vi "Pick&Place_ladder_shih_v4_temp.vi"() -> ()   [LabVIEW 2016]
uses:
  Classes/Controllers/I-O/Copy of NI-DAQ Folder/NI-DAQ.lvclass
  D:/INTT/V1/Classes/Controllers/I-O/Copy of I-O Folder/I-O.lvclass
  Classes/Controllers/Dispenser/Copy of Ultimus V2 Folder/Ultimus V2.lvclass
  <vilib>/Analysis/coordinate.llb/2D Cartesian Coordinate Rotation (Scalar).vi
  <vilib>/Utility/file.llb/Read Delimited Spreadsheet (DBL).vi
  <vilib>/Utility/file.llb/Write Delimited Spreadsheet (DBL).vi
  Classes/Controllers/Motion/Copy of Motion Folder/Motion.lvclass
  Classes/Controllers/Camera/Copy of Controller Folder/Controller.lvclass
  <vilib>/Analysis/NI_AALPro.lvlib
  Classes/Controllers/I-O/Copy of I-O Folder/I-O.lvclass
panel:
  in  "module placing offset":dbl[][](array[numeric])=[[0.0, 0.0, 0.0, 0.0], [0.0, 0.0, 0.0, 0.0]]
  out "after SR":dbl[](array[numeric])
  out "after NL":dbl[](array[numeric])
  out "S chip":dbl[](array[numeric])
  out "N chip":dbl[](array[numeric])
  in  "file path (dialog if empty) 2":path=path "C:/Users/PAGANIS/Desktop/shih cheng wei/OGP/test1-2.txt"
  out "bless from OGP !!! Center of module on stave 3":dbl[](array[numeric])
  out "bless from OGP !! measured stave size  2":dbl[](array[numeric])
  in  "Bless from OGP":bool
  out "FROM Detail !!! Center of module on stave":dbl[](array[numeric])
  out "FROM Detail !! measured stave size":dbl[](array[numeric])
  in  "Align Stave in detail":bool
  in  "check height?":bool
  in  "Uttimus presssure":i64=10
  out "Status":bool
  out "measured HDI top-left position":dbl[][](array[numeric])
  in  "HDI vacuum channel":i32=18
  in  "vacuum":bool=TRUE
  in  "HDI vacuum":bool
  out "measured stave size":dbl[](array[numeric])
  out "Stave mark":dbl[][](array[numeric])
  out "Center of module on stave":dbl[](array[numeric])
  out "Center of HDI from alignment mark":dbl[](array[numeric])
  out "Measured HDI size":dbl[][](array[numeric])
  out "module position on stave":dbl[][](array[numeric])
  in  "Default Stave dimension":dbl[](array[numeric])=[34.0, 472.0, -0.335295, -0.000320234]
  in  "Default Stave upper left mark":dbl[](array[numeric])=[584.376, 675.576, 70.9882, 0.000840064]
  out "Needle parking position":dbl[](array[numeric])
  in  "Uppler / Lower Stave":bool=TRUE
  out "Gantry current position":dbl[](array[numeric])
  in  "READ Position":bool
  in  "Needle Height Compenstation\n(glue gap)":dbl=0.33
  in  "Needle Alignment":bool
  in  "Parking position":dbl[](array[numeric])=[625.0, 625.0, 0.0, 0.01]
  in  "GOTO":bool
  in  "Default Pickup Tool Position":dbl[][](array[numeric])=[[152.226, 682.729, 36.8129, -0.0151898], [700.0, 800.0, 20.0, 0.01]]
  in  "Number of module \nto be assembled":i32=1
  in  "Default HDI alignment \nmark position":dbl[](array[numeric])=[448.322, 976.582, 74.9872, 0.000191129]
  in  "Default HDI size":dbl[](array[numeric])=[24.2437, 231.446, -0.099339, 0.000191129]
  out "# of tasks excuted":i32
  out "module on tray position":dbl[][](array[numeric])
  out "PickupTool \nCenterPosition":dbl[](array[numeric])
  in  "Inititalize":bool
  in  "Pick and place":bool
  in  "Deposit Glue":bool
  in  "Measure Pickup Tools":bool
  in  "Align Stave":bool
  out "default module position on stave":dbl[][](array[numeric])
  in  "Stop":bool
  in  "Measure HDI":bool
  # "Ladder Assembly"
  # "Lower\nmodule"
  # "Upper\nmodule"
  # "Sensor 0.32 -> 200 micron glue thickness\nChips 0.37-> 140 micron glue thickness"
  # "ACTIONS"
  # "Stave infomation"
  # "Module infomation"
  # "Pick and Place"
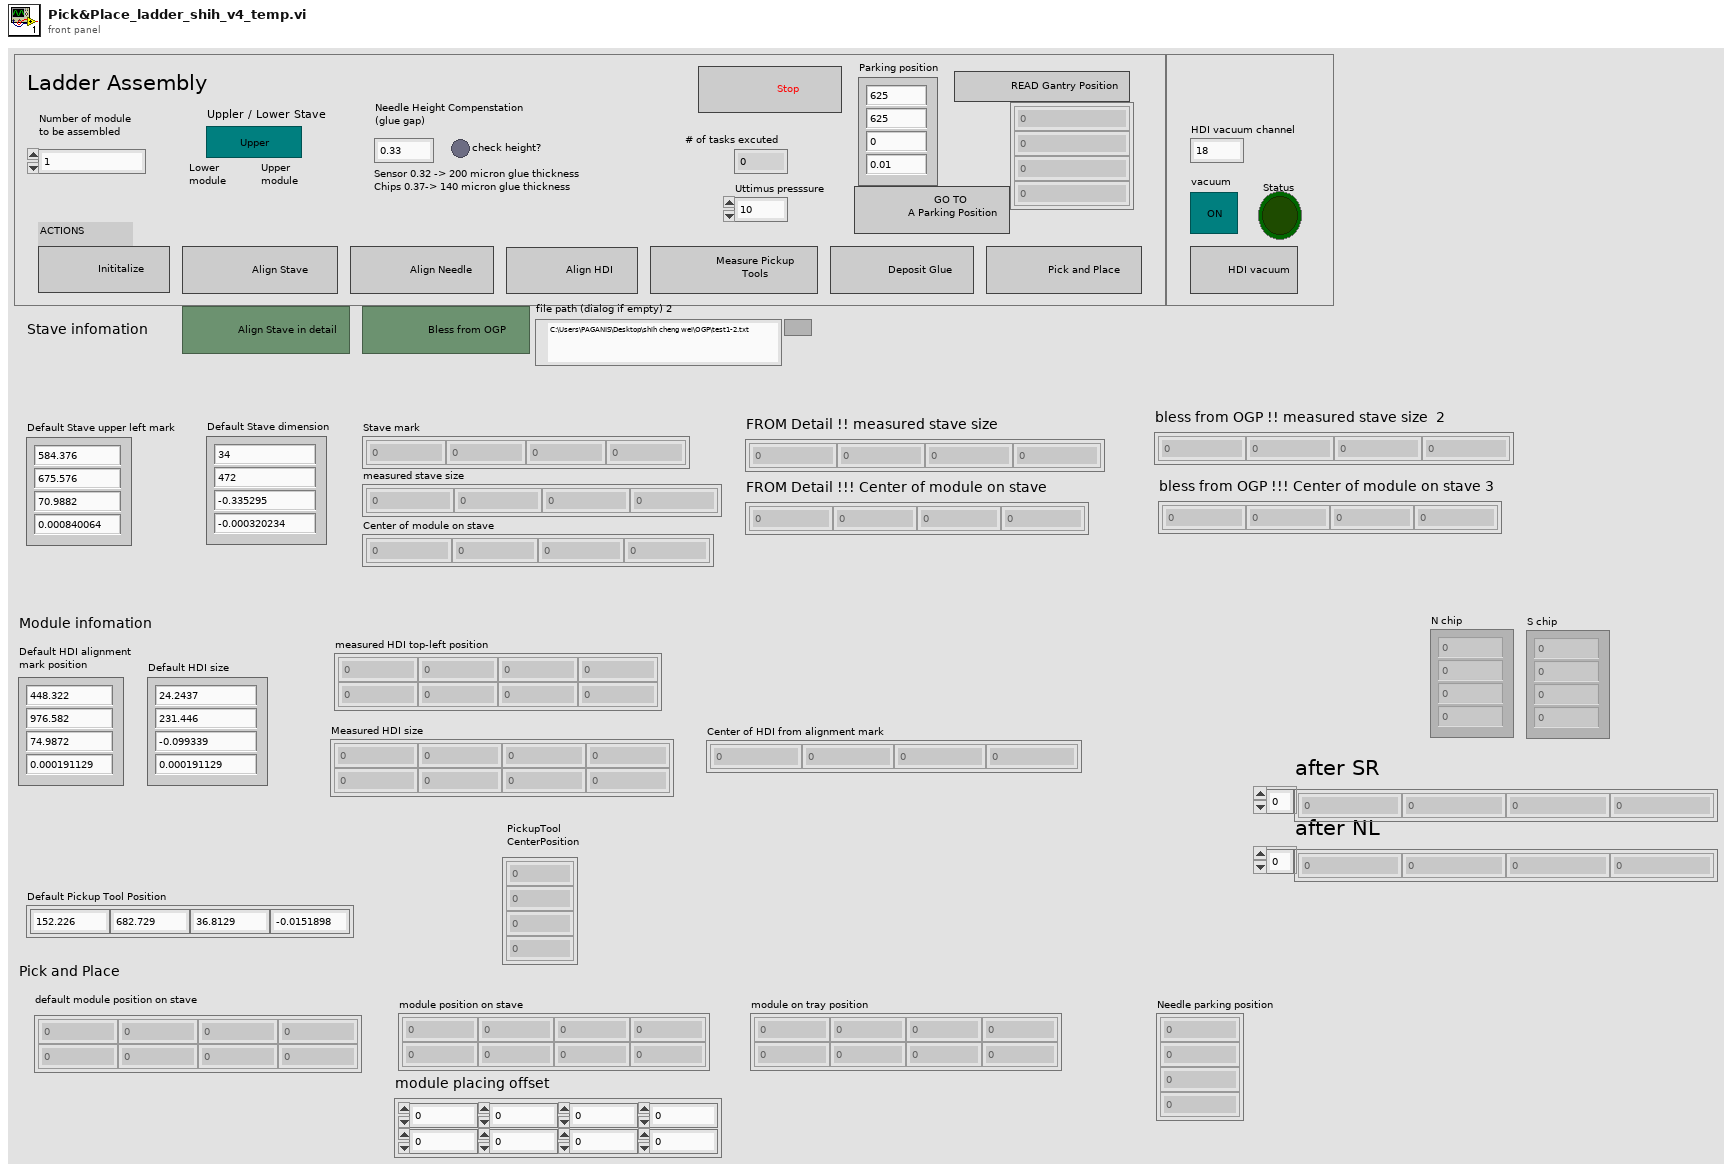
[diagram p1: front panel]
types:
  T1 = typedef "Controller.lvclass/Controllers.ctl" = cluster{"Copy of Motion.lvclass":refnum<class "Motion.lvclass">, "Copy of I-O.lvclass":refnum<class "I-O.lvclass">, "Copy of Dispenser.lvclass":refnum<class "Dispenser.lvclass">}
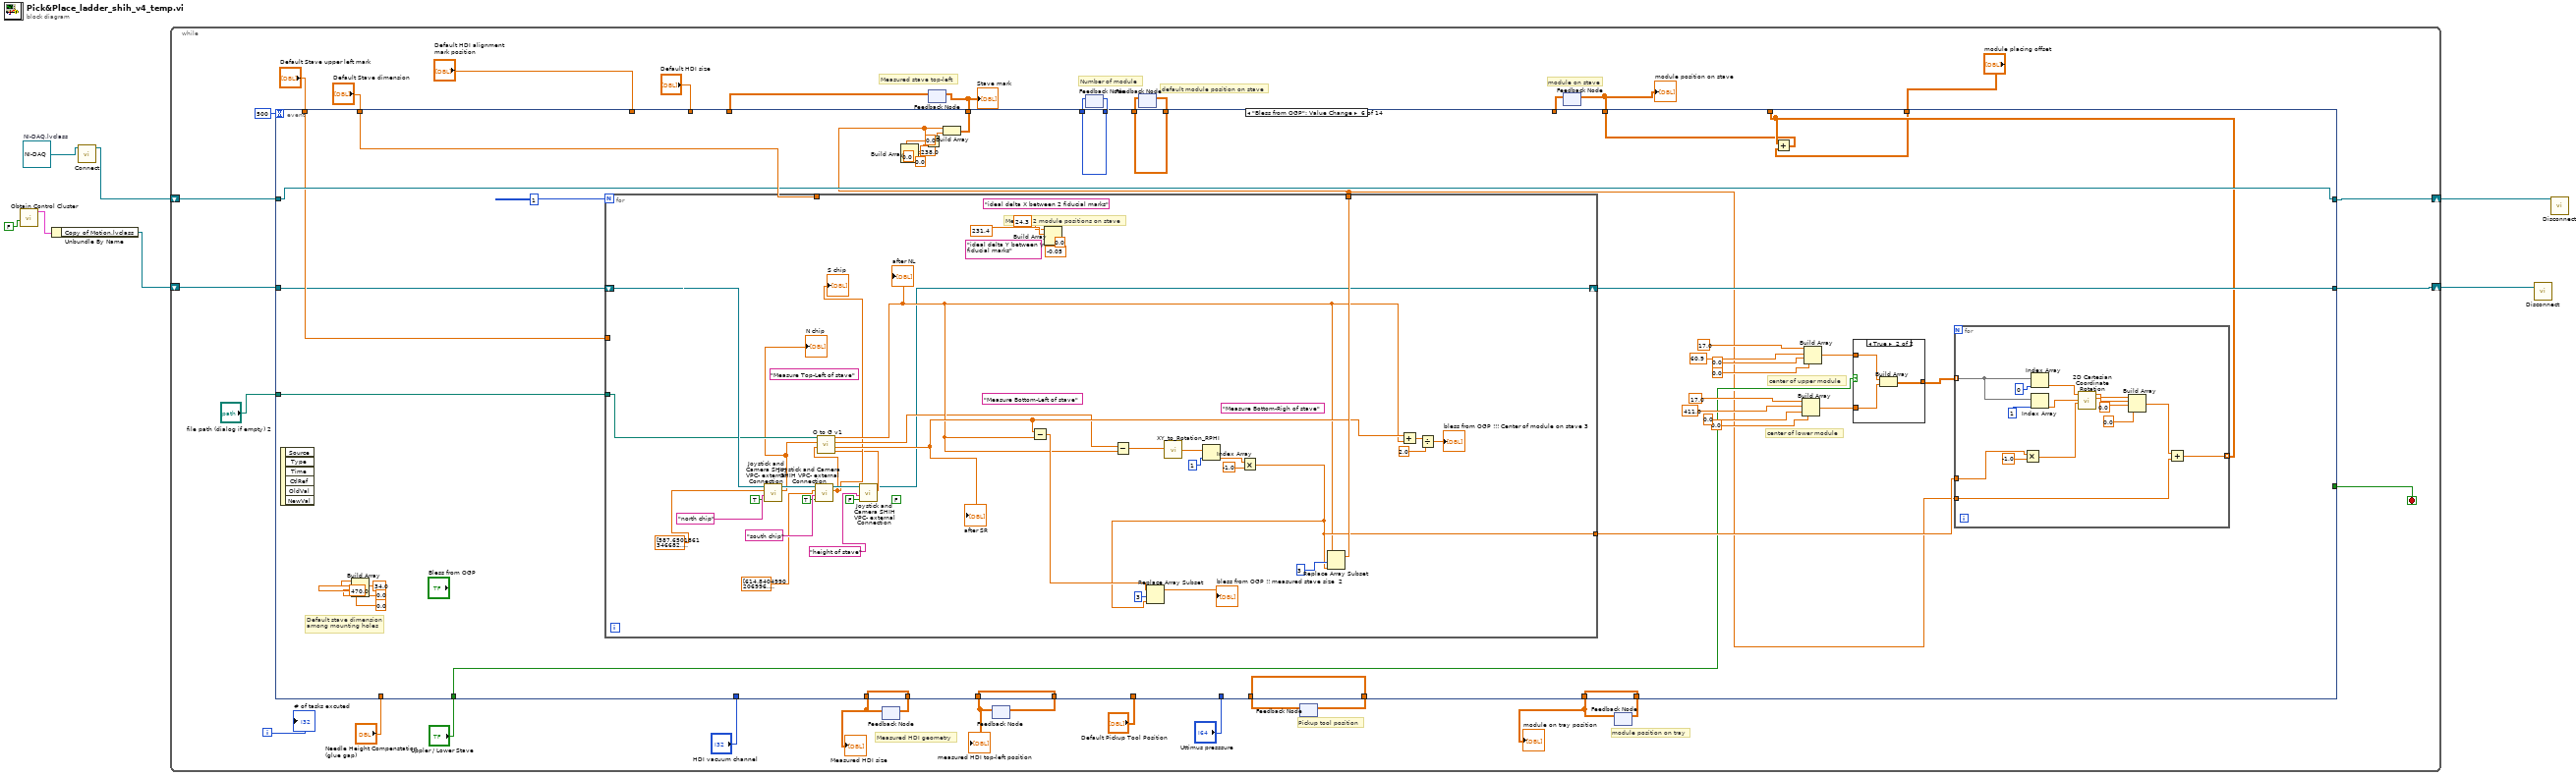
[diagram p0: block diagram]
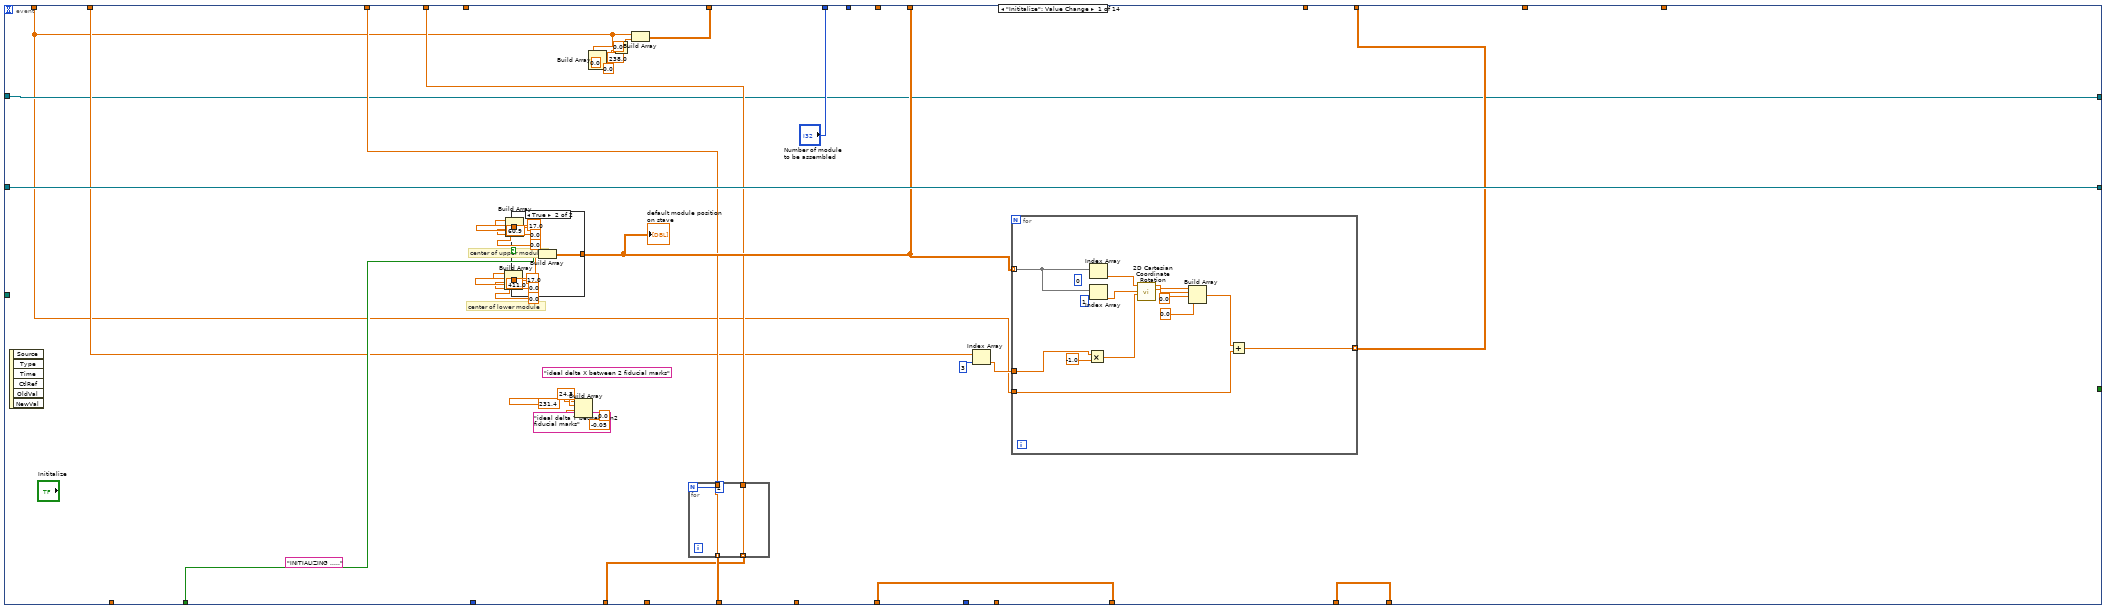
[diagram p2: hidden frame]
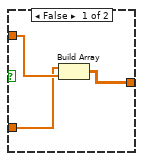
[diagram p3: hidden frame]
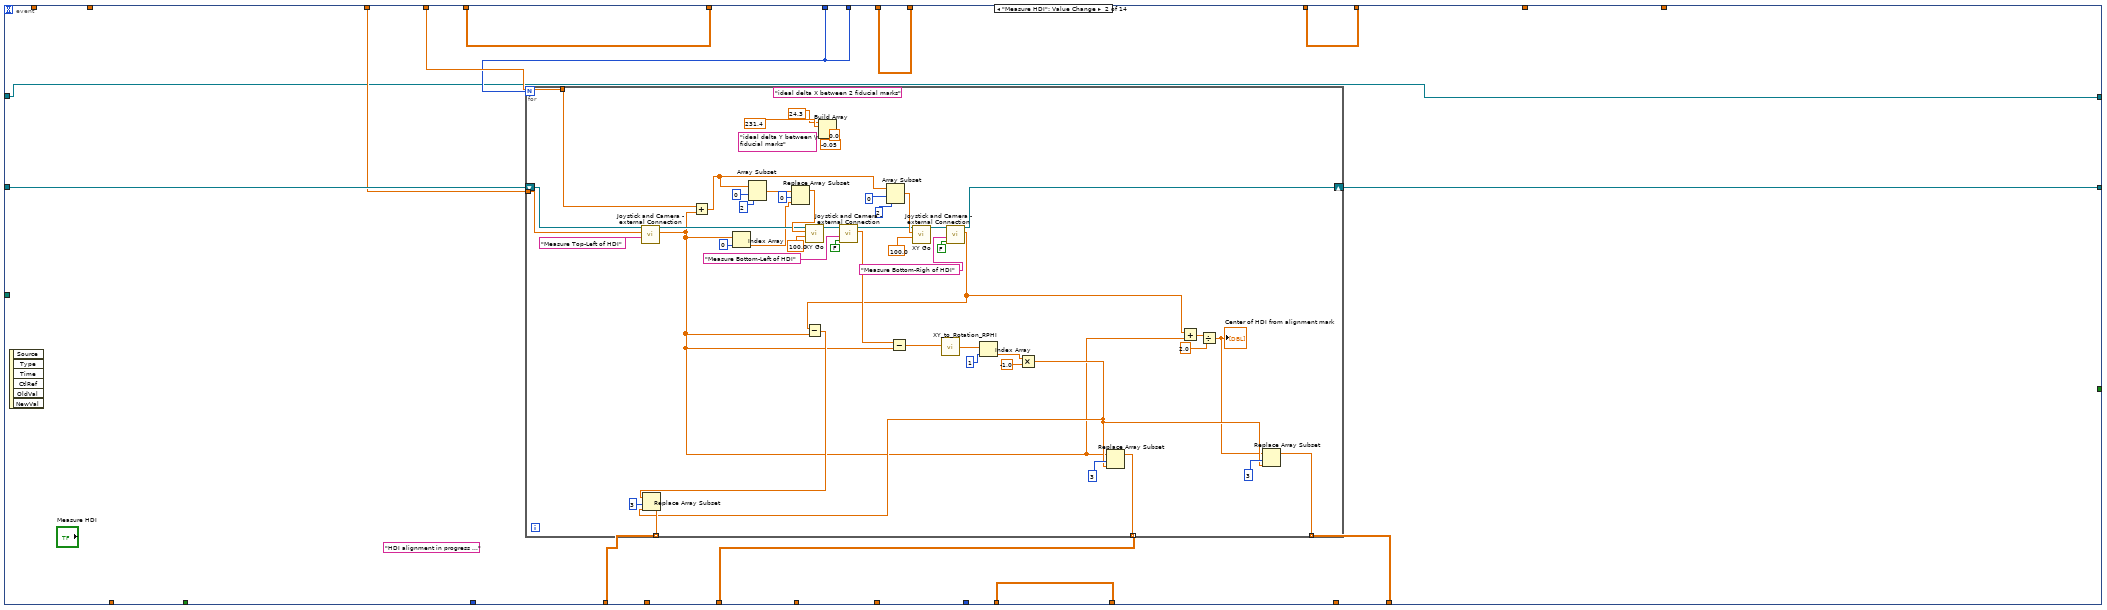
[diagram p4: hidden frame]
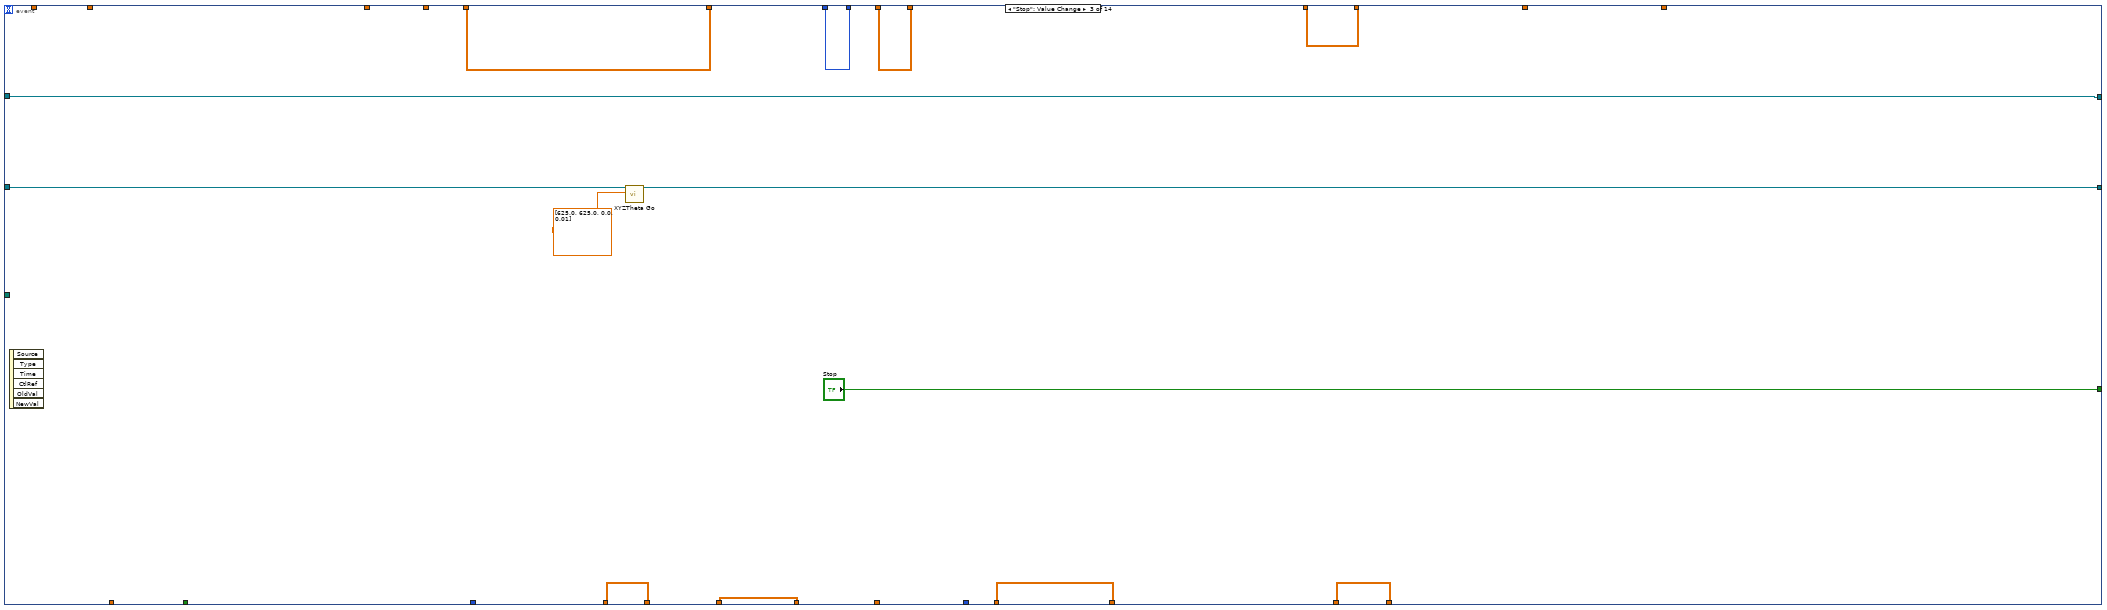
[diagram p5: hidden frame]
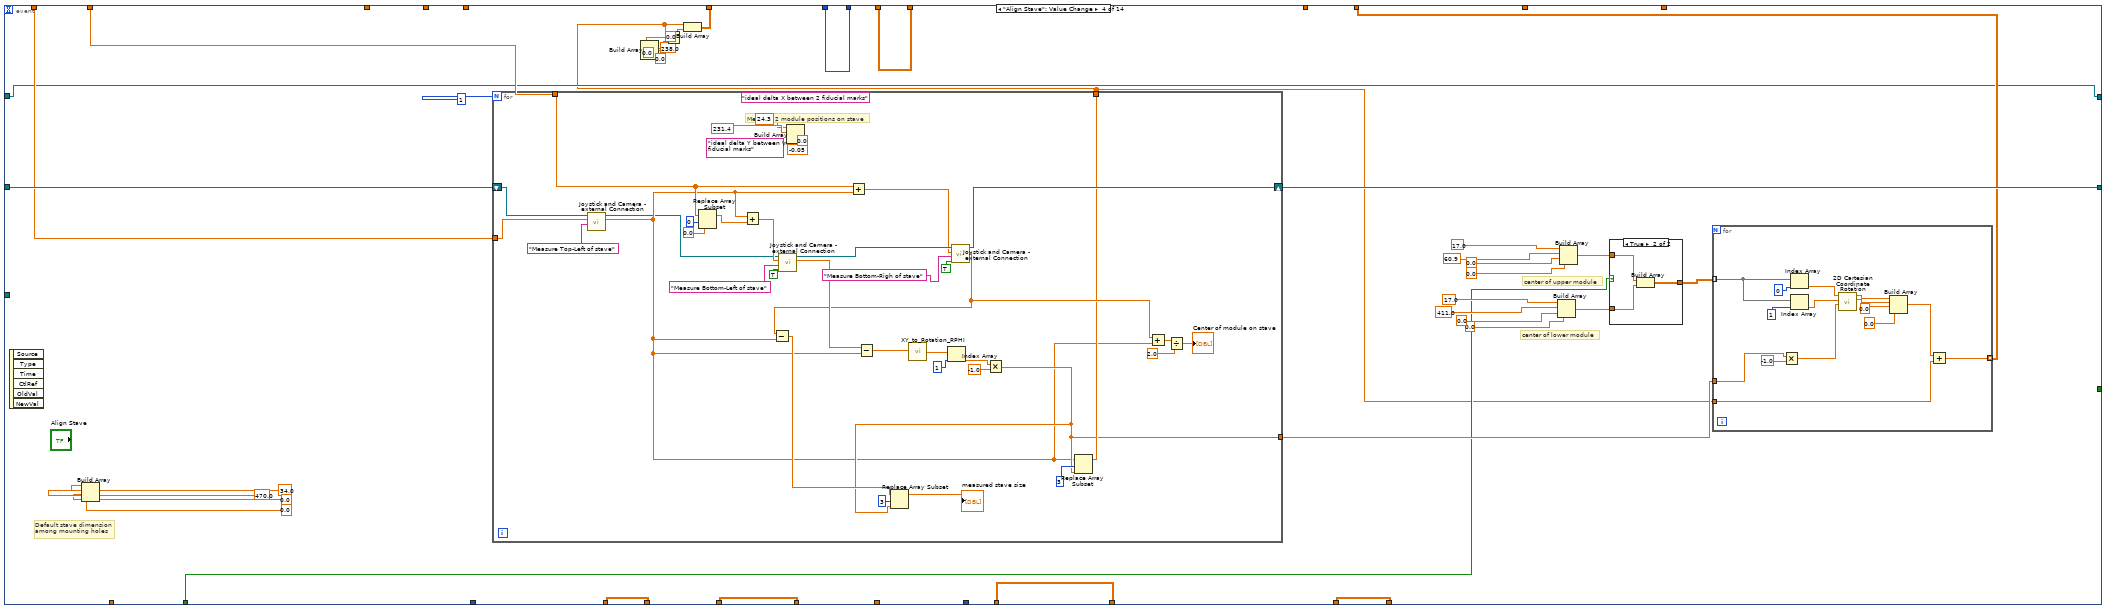
[diagram p6: hidden frame]
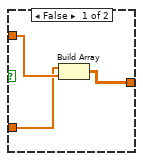
[diagram p7: hidden frame]
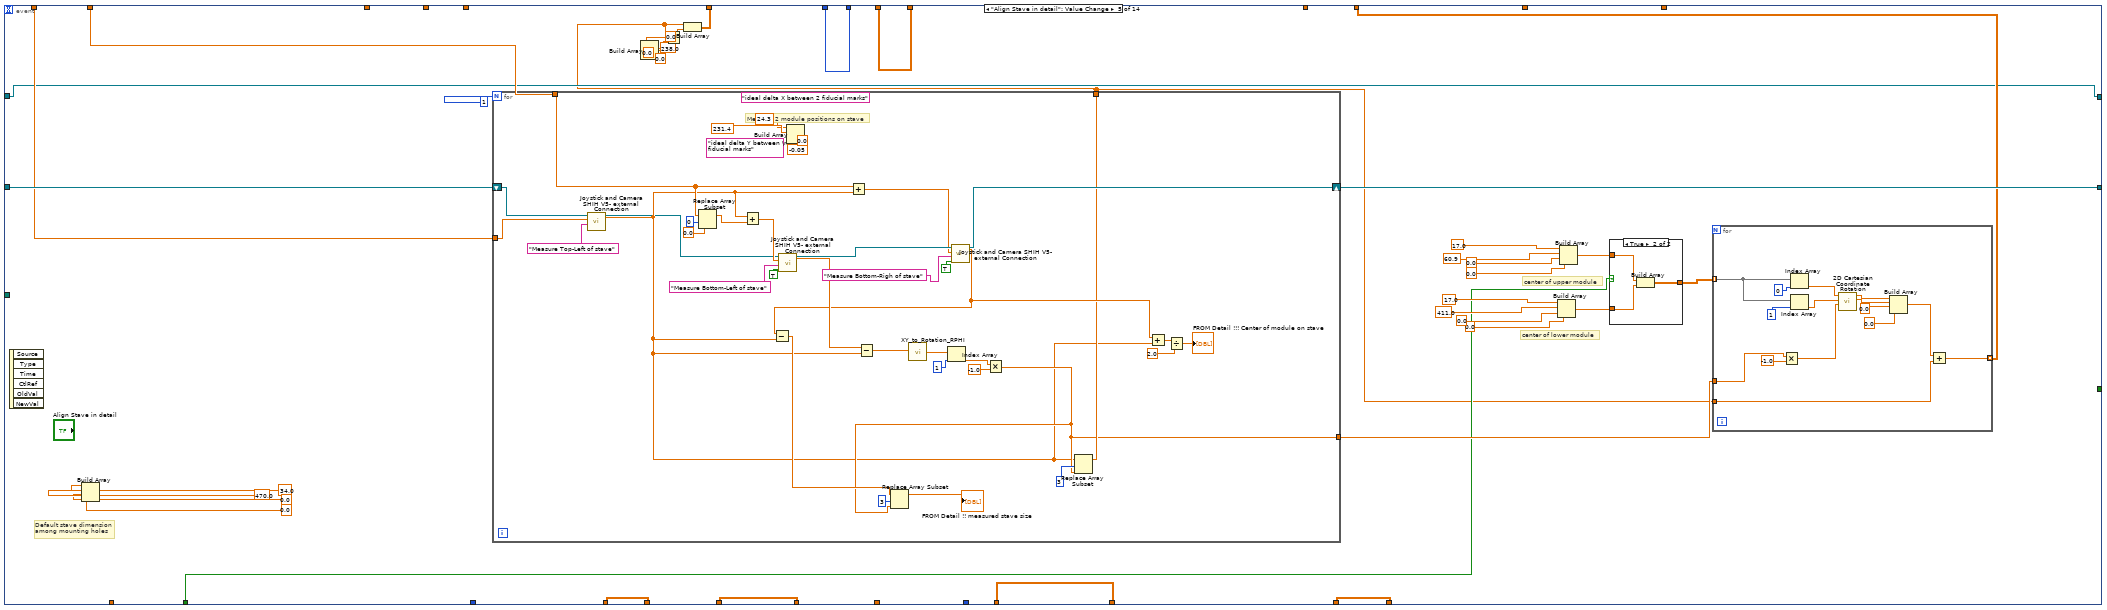
[diagram p8: hidden frame]
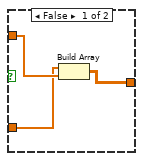
[diagram p9: hidden frame]
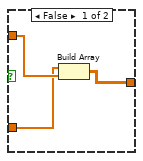
[diagram p10: hidden frame]
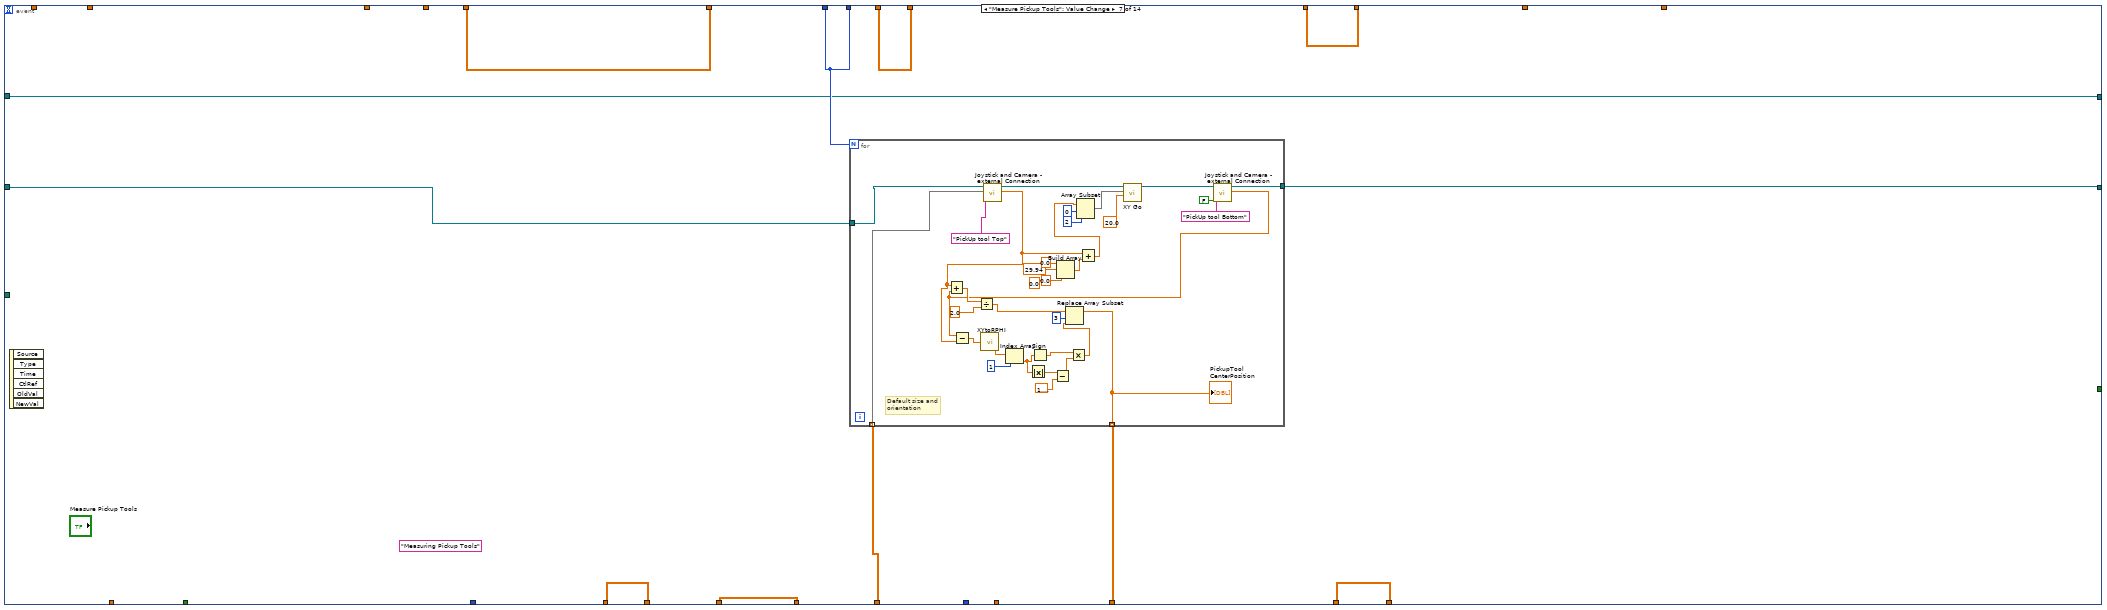
[diagram p11: hidden frame]
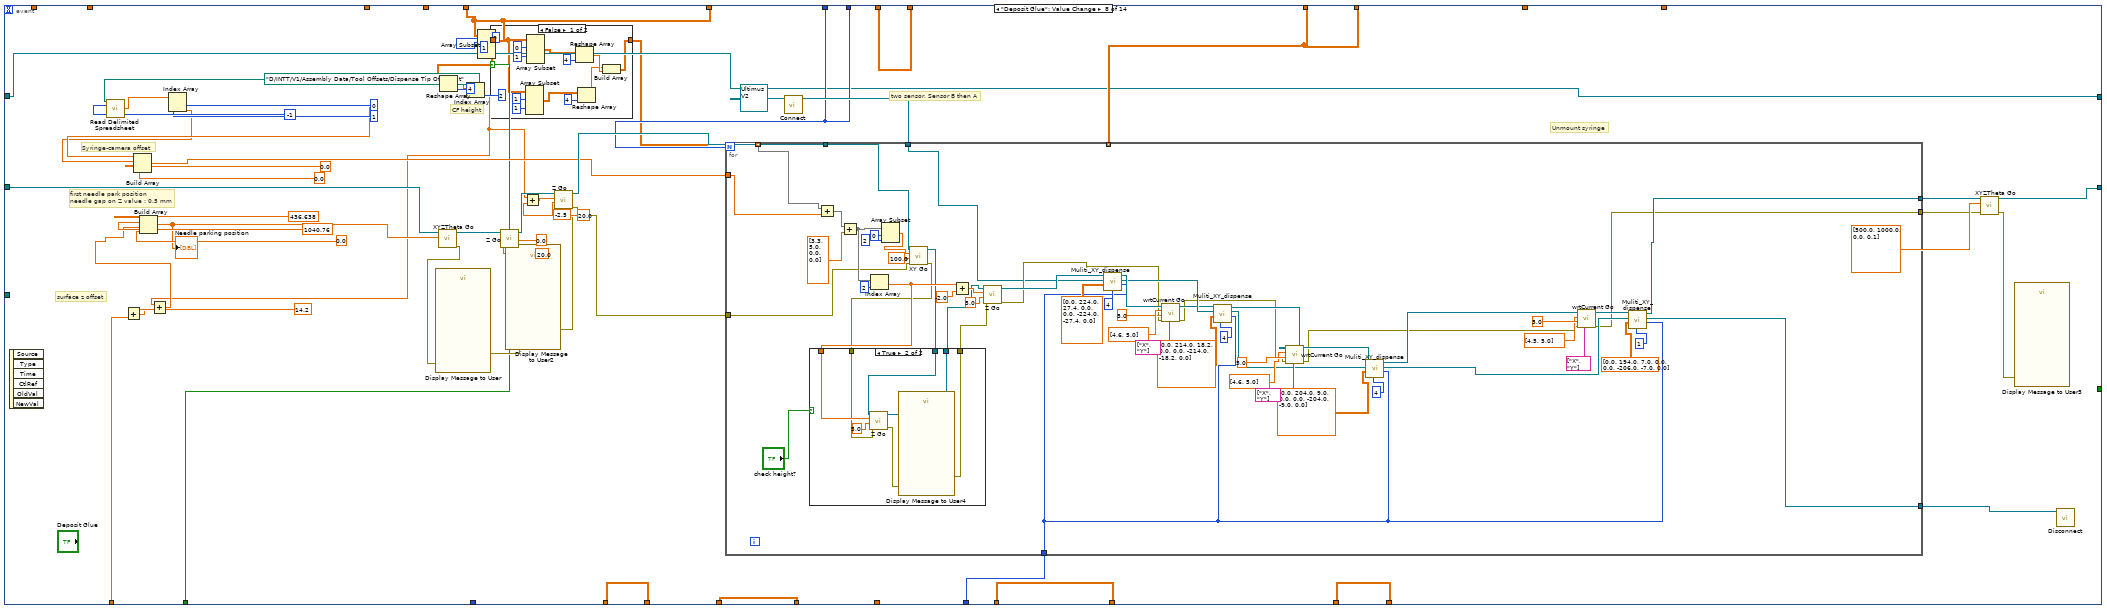
[diagram p12: hidden frame]
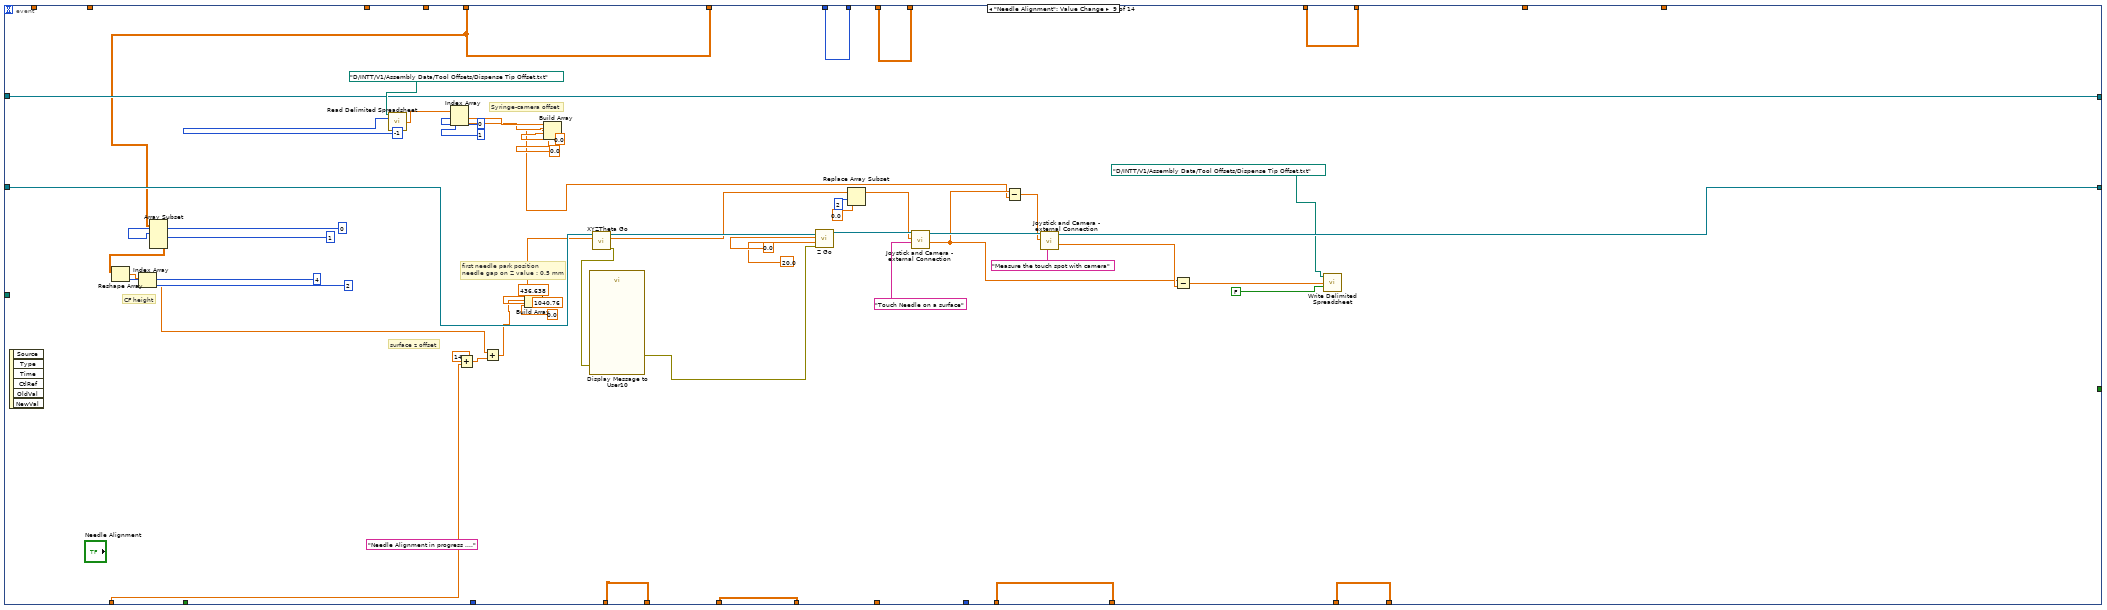
[diagram p15: hidden frame]
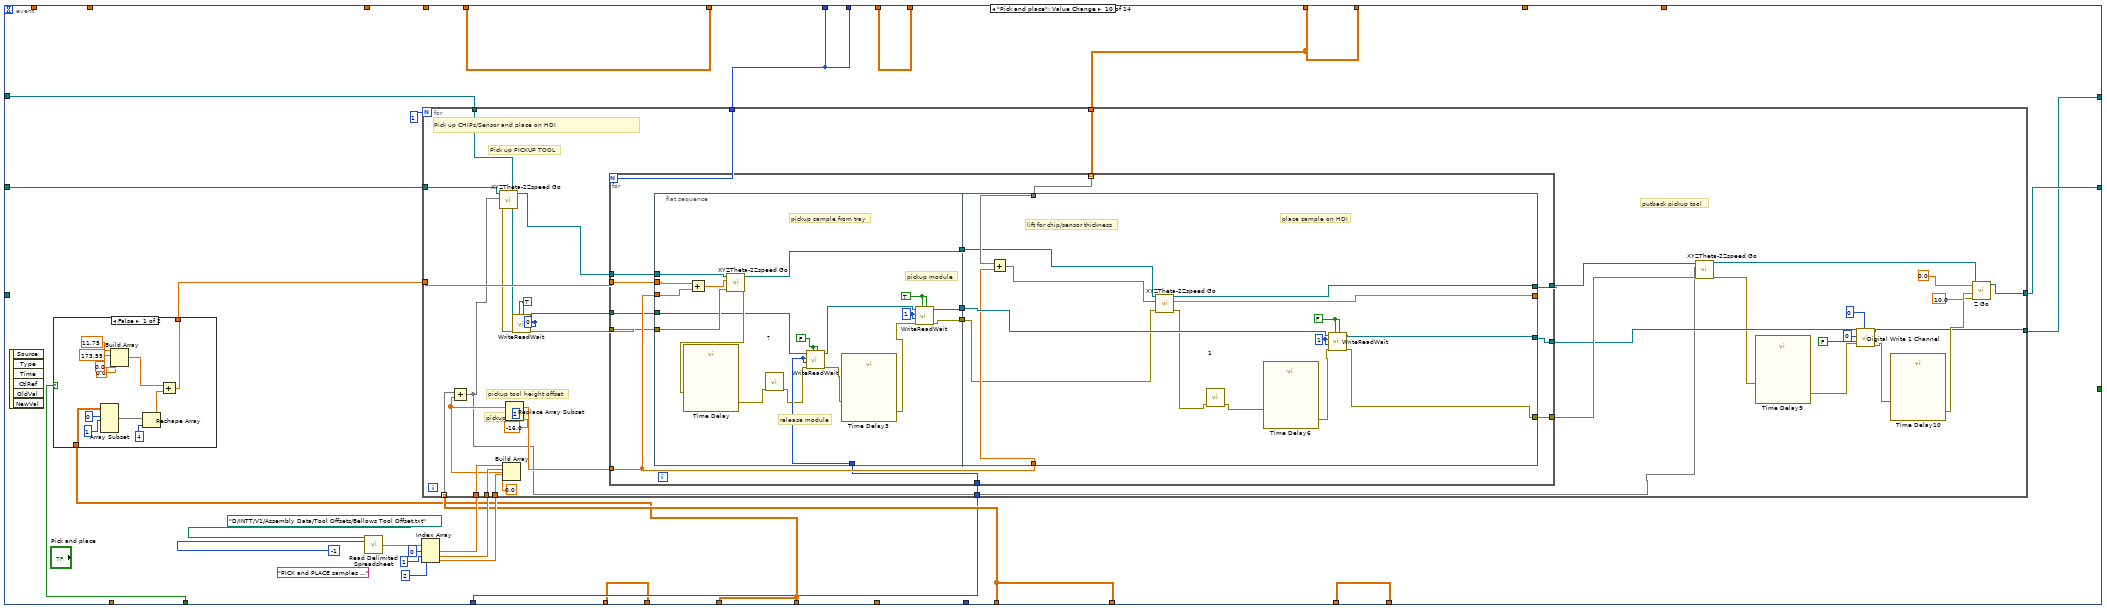
[diagram p16: hidden frame]
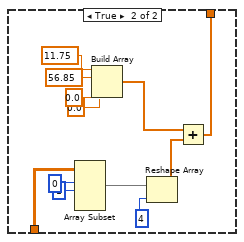
[diagram p17: hidden frame]
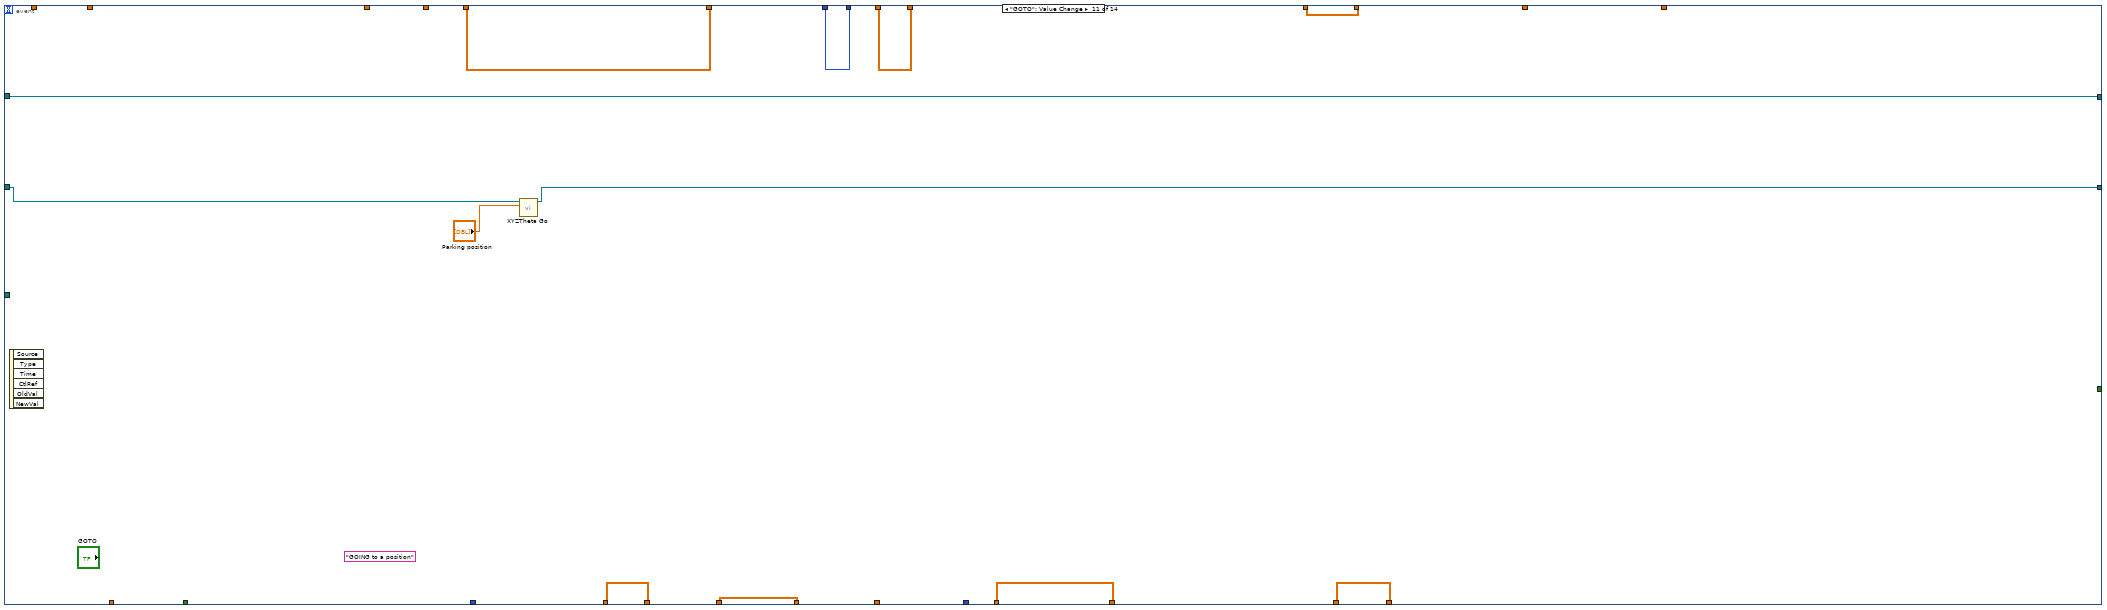
[diagram p18: hidden frame]
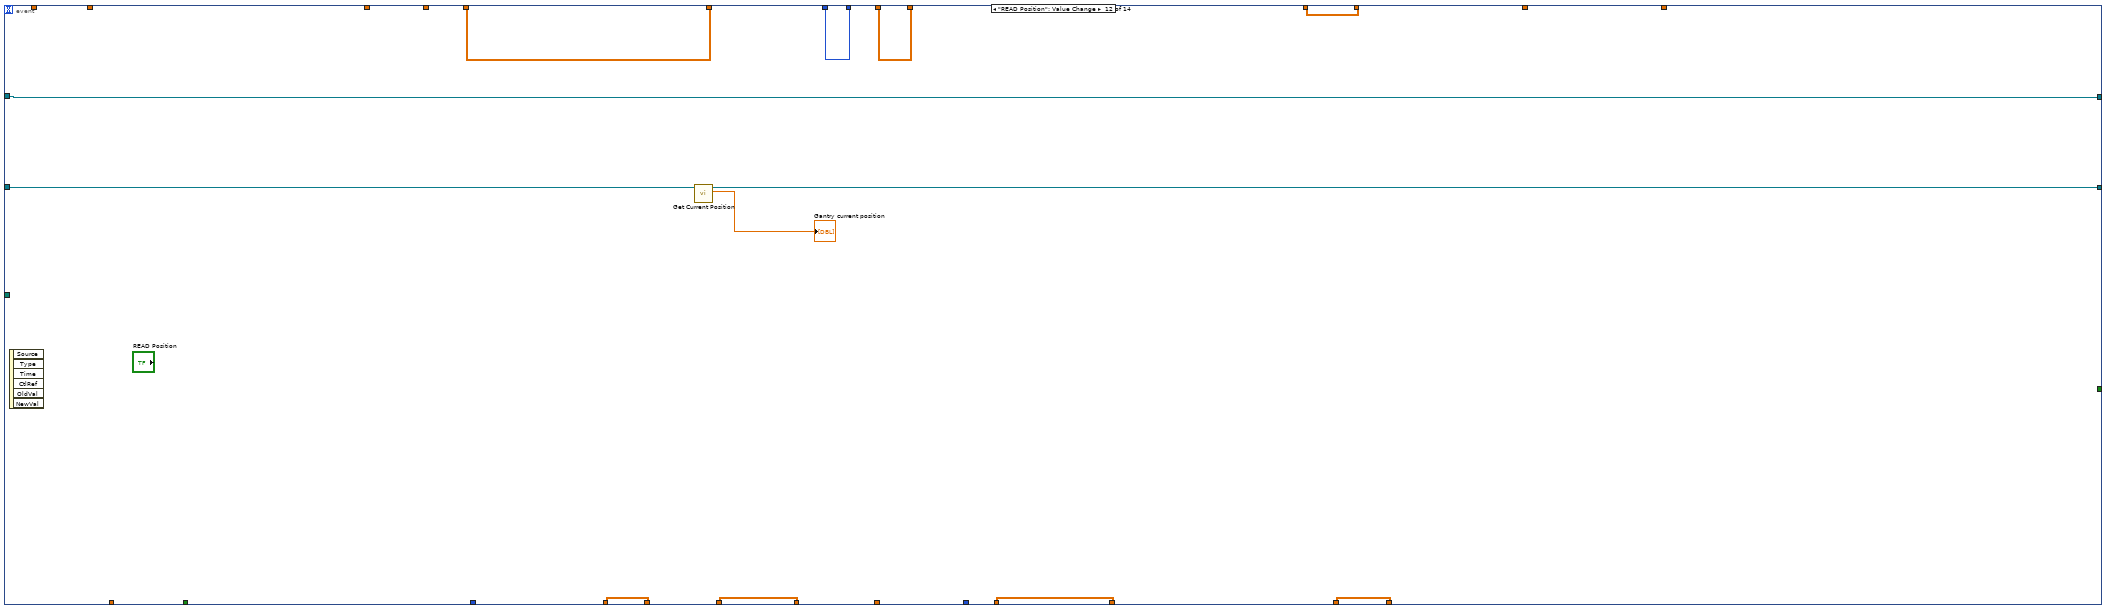
[diagram p19: hidden frame]
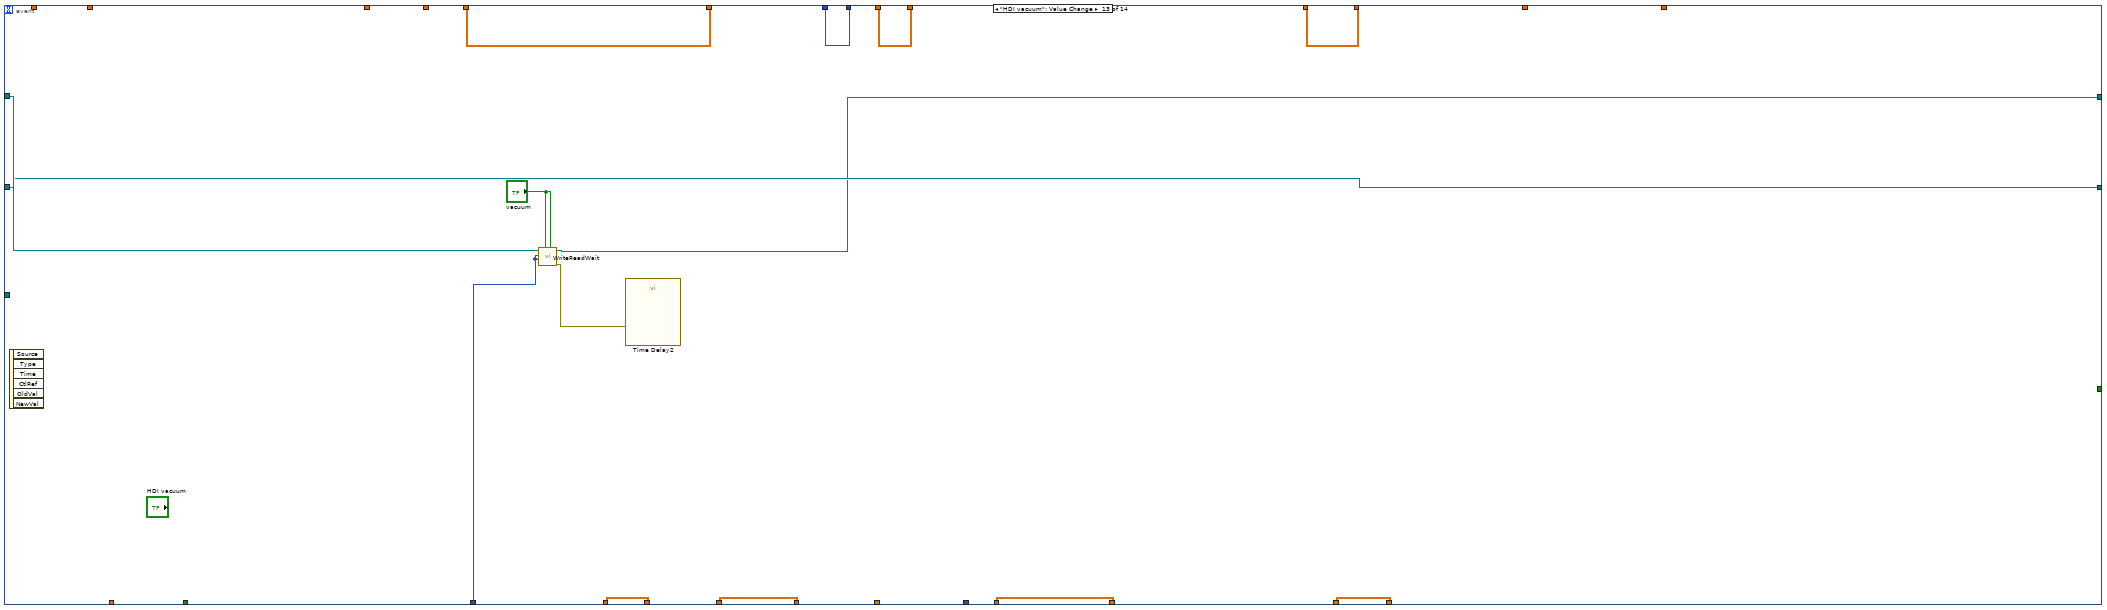
[diagram p20: hidden frame]
diagram:
  w3 = refnum<class "NI-DAQ.lvclass"> refnum  # NI-DAQ.lvclass
  n1 = call "Obtain Control Cluster.vi"("I/O"=FALSE) -> ("Control Out"=w7:T1)  [unwired: 10 in]
  n2 = Unbundle By Name(w7) -> ("Copy of Motion.lvclass"=w5:refnum<class "Motion.lvclass">)
  n3 = call-dynamic "Connect.vi"("NI-DAQ in"=w3) -> ("NI-DAQ out"=w2:refnum<class "NI-DAQ.lvclass">)  [unwired: 9 in, 1 out]
  n4 = while {
    shift-right: [w34] -> w4
    shift-left: w5 -> [w41]
    shift-right: [w13] -> w1
    shift-left: w2 -> [w17]
    i -> [w33]
    stop <- w40 stop-if-true
    # "default module position on stave"
    # "Pickup tool position"
    # "Number of module"
    # "Measured HDI geometry"
    # "module position on tray"
    # "Measured stave top-left"
    # "module on stave"
    n5 = feedback #1() -> (w38:dbl[][])  [unwired: 1 in]
    n6 = feedback #2() -> (w39:dbl[][])  [unwired: 1 in]
    n7 = feedback #3() -> (w14:dbl[][])  [unwired: 1 in]
    n8 = feedback #4() -> (w32:i32)  [unwired: 1 in]
    n9 = feedback #5() -> (w27:dbl[][])  [unwired: 1 in]
    n10 = feedback #6() -> (w35:dbl[][])  [unwired: 1 in]
    n11 = feedback #7() -> (w21:dbl[][])  [unwired: 1 in]
    n12 = feedback #8() -> (w25:dbl[][])  [unwired: 1 in]
    "module on tray position" <- w25
    n13 = event shown="[5] \"Bless from OGP\": Value Change" {
      selector: _ -> [_ _ _ _ _ _ _ _ _ _ _ _ _ _]
      dyn-events: _ -> [_ _ _ _ _ _ _ _ _ _ _ _ _ _]
      timeout: 500 -> [_ _ _ _ _ _ _ _ _ _ _ _ _ _]
      tunnel: w41 -> [w75 w114 w176 w206 w302 w372 w479 w552 w686 w730 w844 w862 w864 w885]
      tunnel: [_ _ "Stop" _ _ _ _ _ _ _ _ _ _ _] -> w40
      tunnel: [w42 w108 w171 w177 w273 w375 w474 w514 w652 w708 w850 w858 w872 w884] -> w18
      tunnel: w39 -> [_ w108 w171 _ _ _ w474 w514 w652 w708 w850 w858 w872 w884]
      tunnel: [w52 w106 w170 w202 w298 w399 w473 w538 w689 w711 w847 w857 w866 w882] -> w19
      tunnel: w38 -> [_ _ w170 w202 w298 w399 w473 w538 w689 w711 w847 w857 w866 w882]
      tunnel: w32 -> [_ w104 w173 w207 w303 w402 w470 w541 w691 w715 w849 w859 w870 w877]
      tunnel: [w57 w105 w168 w209 w305 w404 w472 w540 w687 w718 w845 w855 w868 w879] -> w37
      tunnel: w25 -> [w57 _ w168 w209 w305 w404 w472 w540 w687 w718 w845 w855 w868 w879]
      tunnel: [w73 w109 w169 w214 w310 w409 w478 w539 w688 w719 w846 w856 w867 w880] -> w36
      tunnel: w35 -> [_ w109 w169 w214 w310 w409 _ w539 w688 w719 w846 w856 w867 w880]
      tunnel: [w75 w113 w174 w203 w299 w400 w477 w542 w678 w720 w842 w861 w864 w885] -> w34
      tunnel: ["Number of module \nto be assembled" w104 w173 w207 w303 w402 w470 w541 w691 w715 w849 w859 w870 w877] -> w31
      tunnel: "Default HDI alignment \nmark position" -> [w55 w112 _ _ _ _ _ _ _ _ _ _ _ _]
      tunnel: "Default HDI size" -> [w54 w111 _ _ _ _ _ _ _ _ _ _ _ _]
      tunnel: [w62 w110 w172 w208 w304 w403 w475 w537 w690 w717 w848 w860 w871 w883] -> w28
      tunnel: w27 -> [_ w110 w172 w208 w304 w403 w475 w537 w690 w717 w848 w860 w871 w883]
      tunnel: "Default Pickup Tool Position" -> [w73 _ _ _ _ _ w476 _ _ _ _ _ _ _]
      tunnel: "Uppler / Lower Stave" -> [w58 _ _ w187 w283 w384 _ w522 _ w706 _ _ _ _]
      tunnel: "Default Stave upper left mark" -> [w43 _ _ w205 w301 w374 _ _ _ _ _ _ _ _]
      tunnel: "Default Stave dimension" -> [w51 _ _ w204 w300 w401 _ _ _ _ _ _ _ _]
      tunnel: [w59 w107 w166 w186 w282 w369 w471 w536 w669 w707 w840 w852 w869 w878] -> w20
      tunnel: w21 -> [_ w107 w166 _ _ _ w471 w536 w669 w707 w840 w852 w869 w878]
      tunnel: w17 -> [w50 w102 w164 w185 w281 w383 w468 w531 w667 w714 w839 w851 w876 w888]
      tunnel: [w50 w102 w164 w185 w281 w383 w468 w531 w667 w713 w839 w851 w863 w886] -> w13
      tunnel: "HDI vacuum channel" -> [_ _ _ _ _ _ _ _ _ w712 _ _ w873 w887]
      tunnel: [w53 w103 w165 w201 w297 w398 w469 w532 w668 w710 w841 w853 w865 w881] -> w15
      tunnel: w14 -> [_ _ w165 w201 w297 w398 w469 w532 w668 w710 w841 w853 w865 w881]
      tunnel: "Needle Height Compenstation\n(glue gap)" -> [_ _ _ _ _ _ _ w524 w660 _ _ _ _ _]
      tunnel: "Uttimus presssure" -> [_ _ _ _ _ _ _ w523 _ _ _ _ _ _]
      tunnel: "file path (dialog if empty) 2" -> [_ _ _ _ _ w373 _ _ _ _ _ _ _ _]
      tunnel: [_ _ _ _ _ w371 _ _ _ _ _ _ _ _] -> _
      tunnel: "module placing offset" -> [_ _ _ _ _ w370 _ _ _ _ _ _ _ _]
      event "Inititalize": Value Change {
        (unwired) "INITIALIZING ....." ("String")
        (unwired) "ideal delta Y between \n2 fiducial marks"
        (unwired) "ideal delta X between 2 fiducial marks"
        # "center of lower module"
        # "center of upper module"
        n14 = event-data() -> ()  [unwired: 1 in, 6 out]
        n15 = Build Array(17.0 ("element"), 411.0 ("element"), 0.0 ("element"), 0.0 ("element")) -> (w63:dbl[])
        n16 = Build Array(17.0 ("element"), 60.9 ("element"), 0.0 ("element"), 0.0 ("element")) -> (w64:dbl[])
        n17 = case shown="True" w58 {
          tunnel: w64 -> [w84 w87]
          tunnel: w63 -> [w83 w86]
          tunnel: [w82 w85] -> w62
          frame False {
            n18 = Build Array(w83, w84) -> (w82:dbl[][])
          }
          frame True {
            n19 = Build Array(w87, w86) -> (w85:dbl[][])
          }
        }
        "default module position on stave" <- w62
        n20 = Build Array(24.3 ("y"), 231.4 ("y"), 0.0 ("element"), -0.05 ("element")) -> ()  [unwired: 1 out]
        n21 = Build Array(0.0 ("element"), 238.0 ("element"), 0.0 ("element"), 0.0 ("element")) -> (w45:dbl[])
        n22 = Add(x=w43, y=w45) -> (x+y=w44:dbl[])
        n23 = Build Array(w43, w44) -> (w42:dbl[][])
        n24 = for {
          N: 2 -> [_]
          tunnel: w55 -> [w81]
          tunnel: [w81] -> w53 mode=indexing
          tunnel: w54 -> [w80]
          tunnel: [w80] -> w52 mode=indexing
        }
        n25 = Index Array(array=w51, index=3) -> (element=w60:dbl)
        n26 = for {
          tunnel: w62 -> [w95] mode=indexing
          tunnel: w60 -> [w89]
          tunnel: w43 -> [w94]
          tunnel: [w92] -> w59 mode=indexing
          (unwired) 0 ("index")
          n27 = Multiply(x=w89, y=-1.0) -> (x*y=w90:dbl)
          n28 = Index Array(array=w95) -> (element=w98:dbl)  [unwired: 1 in]
          n29 = Index Array(array=w95, index=1) -> (element=w97:dbl)
          n30 = call-poly <vilib>:"2D Cartesian Coordinate Rotation.vi"("theta"=w90, "y"=w97, "x"=w98) -> ("y out"=w100:dbl, "x out"=w99:dbl)  [unwired: 6 in, 1 out]
          n31 = Build Array(w99, w100, 0.0 ("element"), 0.0 ("element")) -> (w93:dbl[])
          n32 = Add(x=w93, y=w94) -> (x+y=w92:dbl[])
        }
      }
      event "Measure HDI": Value Change {
        (unwired) "HDI alignment in progress ..." ("String")
        n33 = event-data() -> ()  [unwired: 1 in, 6 out]
        n34 = for {
          N: w104 -> [_]
          tunnel: w111 -> [w126]
          shift-right: [w123] -> w113
          shift-left: w114 -> [w124]
          tunnel: w112 -> [w125]
          tunnel: [w160] -> w103 mode=indexing
          tunnel: [w159] -> w106 mode=indexing
          tunnel: [w116] -> w105 mode=indexing
          (unwired) "ideal delta Y between \n2 fiducial marks"
          (unwired) "ideal delta X between 2 fiducial marks"
          n35 = call "Joystick and Camera - external Connection.vi"("Motion in"=w124, "XYZTheta"=w125, "Measurement Point"="Measure Top-Left of HDI") -> ("Motion out"=w139:refnum<class "Motion.lvclass">, "Sum"=w115:dbl[])  [unwired: 4 in, 2 out]
          n36 = Add(x=w126, y=w115) -> (x+y=w143:dbl[])
          n37 = Index Array(array=w115, index=0) -> (element=w130:dbl)
          n38 = Array Subset(array=w143, index=0, length=2) -> (w142:dbl[])
          n39 = Replace Array Subset(array=w142, new element=w130, index=0) -> (w140:dbl[])
          n40 = call-dynamic "XY Go.vi"("Speed"=100.0, "XY"=w140, "Motion in"=w139) -> ("Motion out"=w147:refnum<class "Motion.lvclass">)  [unwired: 7 in, 1 out]
          n41 = Build Array(24.3 ("y"), 231.4 ("y"), 0.0 ("element"), -0.05 ("element")) -> ()  [unwired: 1 out]
          n42 = call "Joystick and Camera - external Connection.vi"("Motion in"=w147, "Measurement Point"="Measure Bottom-Left of HDI", "Inital GO"=FALSE) -> ("Motion out"=w138:refnum<class "Motion.lvclass">, "Sum"=w129:dbl[])  [unwired: 4 in, 2 out]
          n43 = Array Subset(array=w143, index=0, length=2) -> (w153:dbl[])
          n44 = Subtract(x=w129, y=w115) -> (x-y=w137:dbl[])
          n45 = call-dynamic "XY Go.vi"("Speed"=100.0, "XY"=w153, "Motion in"=w138) -> ("Motion out"=w157:refnum<class "Motion.lvclass">)  [unwired: 7 in, 1 out]
          n46 = call "XY_to_Rotation_RPHI.vi"("X-Y"=w137) -> ("r-phi"=w133:dbl[])
          n47 = call "Joystick and Camera - external Connection.vi"("Motion in"=w157, "Measurement Point"="Measure Bottom-Righ of HDI", "Inital GO"=FALSE) -> ("Motion out"=w123:refnum<class "Motion.lvclass">, "Sum"=w120:dbl[])  [unwired: 4 in, 2 out]
          n48 = Subtract(x=w120, y=w115) -> (x-y=w121:dbl[])
          n49 = Index Array(array=w133, index=1) -> (element=w127:dbl)
          n50 = Multiply(x=w127, y=-1.0) -> (x*y=w118:dbl)
          n51 = Replace Array Subset(array=w121, new element=w118, index=3) -> (w159:dbl[])
          n52 = Replace Array Subset(array=w115, new element=w118, index=3) -> (w160:dbl[])
          n53 = Add(x=w120, y=w115) -> (x+y=w162:dbl[])
          n54 = Divide(x=w162, y=2.0) -> (x/y=w117:dbl[])
          "Center of HDI from alignment mark" <- w117
          n55 = Replace Array Subset(array=w117, new element=w118, index=3) -> (w116:dbl[])
        }
      }
      event "Stop": Value Change {
        n56 = event-data() -> ()  [unwired: 1 in, 6 out]
        n57 = call "XYZTheta Go.vi"("XYZTheta In"=dbl[] [625.0, 625.0, 0.0, 0.01], "Motion in"=w176) -> ("Motion out"=w174:refnum<class "Motion.lvclass">)  [unwired: 7 in, 2 out]
      }
      event "Align Stave": Value Change {
        # "center of lower module"
        # "center of upper module"
        # "Default stave dimension\namong mounting holes"
        # "Measure 2 module positions on stave"
        n58 = event-data() -> ()  [unwired: 1 in, 6 out]
        n59 = Build Array(34.0 ("element"), 470.0 ("element"), 0.0 ("element"), 0.0 ("element")) -> ()  [unwired: 1 out]
        n60 = for {
          N: 1 -> [_]
          tunnel: w204 -> [w221]
          shift-right: [w231] -> w203
          shift-left: w206 -> [w232]
          tunnel: w205 -> [w233]
          tunnel: [w226] -> w179
          tunnel: [w224] -> w189
          (unwired) "ideal delta Y between \n2 fiducial marks"
          (unwired) "ideal delta X between 2 fiducial marks"
          n61 = call "Joystick and Camera - external Connection.vi"("Motion in"=w232, "XYZTheta"=w233, "Measurement Point"="Measure Top-Left of stave") -> ("Motion out"=w215:refnum<class "Motion.lvclass">, "Sum"=w217:dbl[])  [unwired: 4 in, 2 out]
          n62 = Replace Array Subset(array=w221, new element=0.0 ("new element/subarray"), index=0) -> (w218:dbl[])
          n63 = Add(x=w217, y=w218) -> (x+y=w216:dbl[])
          n64 = call "Joystick and Camera - external Connection.vi"("Motion in"=w215, "XYZTheta"=w216, "Measurement Point"="Measure Bottom-Left of stave", "Inital GO"=TRUE) -> ("Motion out"=w223:refnum<class "Motion.lvclass">, "Sum"=w236:dbl[])  [unwired: 3 in, 2 out]
          n65 = Build Array(24.3 ("y"), 231.4 ("y"), 0.0 ("element"), -0.05 ("element")) -> ()  [unwired: 1 out]
          n66 = Add(x=w221, y=w217) -> (x+y=w222:dbl[])
          n67 = Subtract(x=w236, y=w217) -> (x-y=w242:dbl[])
          n68 = call "XY_to_Rotation_RPHI.vi"("X-Y"=w242) -> ("r-phi"=w238:dbl[])
          n69 = Index Array(array=w238, index=1) -> (element=w234:dbl)
          n70 = call "Joystick and Camera - external Connection.vi"("Motion in"=w223, "XYZTheta"=w222, "Measurement Point"="Measure Bottom-Righ of stave", "Inital GO"=TRUE) -> ("Motion out"=w231:refnum<class "Motion.lvclass">, "Sum"=w228:dbl[])  [unwired: 3 in, 2 out]
          n71 = Subtract(x=w228, y=w217) -> (x-y=w229:dbl[])
          n72 = Multiply(x=w234, y=-1.0) -> (x*y=w224:dbl)
          n73 = Replace Array Subset(array=w229, new element=w224, index=3) -> (→"measured stave size":dbl[])
          n74 = Replace Array Subset(array=w217, new element=w224, index=3) -> (w226:dbl[])
          n75 = Add(x=w228, y=w217) -> (x+y=w250:dbl[])
          n76 = Divide(x=w250, y=2.0) -> (x/y=→"Center of module on stave":dbl[])
        }
        n77 = Build Array(0.0 ("element"), 238.0 ("element"), 0.0 ("element"), 0.0 ("element")) -> (w180:dbl[])
        n78 = Add(x=w179, y=w180) -> (x+y=w178:dbl[])
        n79 = Build Array(w179, w178) -> (w177:dbl[][])
        n80 = Build Array(17.0 ("element"), 411.0 ("element"), 0.0 ("element"), 0.0 ("element")) -> (w191:dbl[])
        n81 = Build Array(17.0 ("element"), 60.9 ("element"), 0.0 ("element"), 0.0 ("element")) -> (w192:dbl[])
        n82 = case shown="True" w187 {
          tunnel: w192 -> [w269 w272]
          tunnel: w191 -> [w268 w271]
          tunnel: [w267 w270] -> w190
          frame False {
            n83 = Build Array(w268, w269) -> (w267:dbl[][])
          }
          frame True {
            n84 = Build Array(w272, w271) -> (w270:dbl[][])
          }
        }
        n85 = for {
          tunnel: w190 -> [w260] mode=indexing
          tunnel: w189 -> [w255]
          tunnel: w179 -> [w259]
          tunnel: [w257] -> w186 mode=indexing
          n86 = Multiply(x=w255, y=-1.0) -> (x*y=w254:dbl)
          n87 = Index Array(array=w260, index=0) -> (element=w263:dbl)
          n88 = Index Array(array=w260, index=1) -> (element=w262:dbl)
          n89 = call-poly <vilib>:"2D Cartesian Coordinate Rotation.vi"("theta"=w254, "y"=w262, "x"=w263) -> ("y out"=w265:dbl, "x out"=w264:dbl)  [unwired: 6 in, 1 out]
          n90 = Build Array(w264, w265, 0.0 ("element"), 0.0 ("element")) -> (w258:dbl[])
          n91 = Add(x=w258, y=w259) -> (x+y=w257:dbl[])
        }
      }
      event "Align Stave in detail": Value Change {
        # "center of lower module"
        # "center of upper module"
        # "Default stave dimension\namong mounting holes"
        # "Measure 2 module positions on stave"
        n92 = event-data() -> ()  [unwired: 1 in, 6 out]
        n93 = Build Array(34.0 ("element"), 470.0 ("element"), 0.0 ("element"), 0.0 ("element")) -> ()  [unwired: 1 out]
        n94 = for {
          N: 1 -> [_]
          tunnel: w300 -> [w317]
          shift-right: [w327] -> w299
          shift-left: w302 -> [w328]
          tunnel: w301 -> [w329]
          tunnel: [w322] -> w275
          tunnel: [w320] -> w285
          (unwired) "ideal delta Y between \n2 fiducial marks"
          (unwired) "ideal delta X between 2 fiducial marks"
          n95 = call "Joystick and Camera SHIH V5- external Connection.vi"("Motion in"=w328, "XYZTheta"=w329, "Measurement Point"="Measure Top-Left of stave") -> ("final out"=w313:dbl[], "Motion out"=w311:refnum<class "Motion.lvclass">)  [unwired: 5 in, 1 out]
          n96 = Replace Array Subset(array=w317, new element=0.0 ("new element/subarray"), index=0) -> (w314:dbl[])
          n97 = Add(x=w313, y=w314) -> (x+y=w312:dbl[])
          n98 = call "Joystick and Camera SHIH V5- external Connection.vi"("Motion in"=w311, "XYZTheta"=w312, "Measurement Point"="Measure Bottom-Left of stave", "Inital GO"=TRUE) -> ("final out"=w332:dbl[], "Motion out"=w319:refnum<class "Motion.lvclass">)  [unwired: 4 in, 1 out]
          n99 = Build Array(24.3 ("y"), 231.4 ("y"), 0.0 ("element"), -0.05 ("element")) -> ()  [unwired: 1 out]
          n100 = Add(x=w317, y=w313) -> (x+y=w318:dbl[])
          n101 = Subtract(x=w332, y=w313) -> (x-y=w338:dbl[])
          n102 = call "XY_to_Rotation_RPHI.vi"("X-Y"=w338) -> ("r-phi"=w334:dbl[])
          n103 = Index Array(array=w334, index=1) -> (element=w330:dbl)
          n104 = call "Joystick and Camera SHIH V5- external Connection.vi"("Motion in"=w319, "XYZTheta"=w318, "Measurement Point"="Measure Bottom-Righ of stave", "Inital GO"=TRUE) -> ("final out"=w324:dbl[], "Motion out"=w327:refnum<class "Motion.lvclass">)  [unwired: 4 in, 1 out]
          n105 = Subtract(x=w324, y=w313) -> (x-y=w325:dbl[])
          n106 = Multiply(x=w330, y=-1.0) -> (x*y=w320:dbl)
          n107 = Replace Array Subset(array=w325, new element=w320, index=3) -> (→"FROM Detail !! measured stave size":dbl[])
          n108 = Replace Array Subset(array=w313, new element=w320, index=3) -> (w322:dbl[])
          n109 = Add(x=w324, y=w313) -> (x+y=w346:dbl[])
          n110 = Divide(x=w346, y=2.0) -> (x/y=→"FROM Detail !!! Center of module on stave":dbl[])
        }
        n111 = Build Array(0.0 ("element"), 238.0 ("element"), 0.0 ("element"), 0.0 ("element")) -> (w276:dbl[])
        n112 = Add(x=w275, y=w276) -> (x+y=w274:dbl[])
        n113 = Build Array(w275, w274) -> (w273:dbl[][])
        n114 = Build Array(17.0 ("element"), 411.0 ("element"), 0.0 ("element"), 0.0 ("element")) -> (w287:dbl[])
        n115 = Build Array(17.0 ("element"), 60.9 ("element"), 0.0 ("element"), 0.0 ("element")) -> (w288:dbl[])
        n116 = case shown="True" w283 {
          tunnel: w288 -> [w365 w368]
          tunnel: w287 -> [w364 w367]
          tunnel: [w363 w366] -> w286
          frame False {
            n117 = Build Array(w364, w365) -> (w363:dbl[][])
          }
          frame True {
            n118 = Build Array(w368, w367) -> (w366:dbl[][])
          }
        }
        n119 = for {
          tunnel: w286 -> [w356] mode=indexing
          tunnel: w285 -> [w351]
          tunnel: w275 -> [w355]
          tunnel: [w353] -> w282 mode=indexing
          n120 = Multiply(x=w351, y=-1.0) -> (x*y=w350:dbl)
          n121 = Index Array(array=w356, index=0) -> (element=w359:dbl)
          n122 = Index Array(array=w356, index=1) -> (element=w358:dbl)
          n123 = call-poly <vilib>:"2D Cartesian Coordinate Rotation.vi"("theta"=w350, "y"=w358, "x"=w359) -> ("y out"=w361:dbl, "x out"=w360:dbl)  [unwired: 6 in, 1 out]
          n124 = Build Array(w360, w361, 0.0 ("element"), 0.0 ("element")) -> (w354:dbl[])
          n125 = Add(x=w354, y=w355) -> (x+y=w353:dbl[])
        }
      }
      event "Bless from OGP": Value Change {
        # "center of lower module"
        # "center of upper module"
        # "Default stave dimension\namong mounting holes"
        # "Measure 2 module positions on stave"
        n126 = event-data() -> ()  [unwired: 1 in, 6 out]
        n127 = Build Array(34.0 ("element"), 470.0 ("element"), 0.0 ("element"), 0.0 ("element")) -> ()  [unwired: 1 out]
        n128 = for {
          N: 1 -> [_]
          tunnel: w401 -> [_]
          shift-right: [w412] -> w400
          shift-left: w372 -> [w428]
          tunnel: w374 -> [_]
          tunnel: [w431] -> w377
          tunnel: [w429] -> w386
          tunnel: w373 -> [w416]
          (unwired) FALSE ("Inital GO")
          (unwired) "Measure Bottom-Righ of stave" ("Measurement Point")
          (unwired) "Measure Bottom-Left of stave" ("Measurement Point")
          (unwired) "Measure Top-Left of stave" ("Measurement Point")
          (unwired) "ideal delta Y between \n2 fiducial marks"
          (unwired) "ideal delta X between 2 fiducial marks"
          n129 = call "Joystick and Camera SHIH VPC- external Connection.vi"("Motion in"=w428, "XYZTheta"=dbl[] [587.6501861346682, 659.8354057217969, 70.1155335060548, 0.010000094994154989] ("N chip"), "Measurement Point"="north chip", "Inital GO"=TRUE) -> ("Motion out"=w425:refnum<class "Motion.lvclass">, "Sum"=w415:dbl[])  [unwired: 3 in, 2 out]
          "N chip" <- w415
          n130 = call "Joystick and Camera SHIH VPC- external Connection.vi"("Motion in"=w425, "XYZTheta"=dbl[] [614.8404990206996, 1158.7590823829282, 70.34521582498871, 0.010000670236950445] ("S chip"), "Measurement Point"="south chip", "Inital GO"=TRUE) -> ("Motion out"=w424:refnum<class "Motion.lvclass">, "Sum"=w414:dbl[])  [unwired: 3 in, 2 out]
          "S chip" <- w414
          n131 = call "Joystick and Camera SHIH VPC- external Connection.vi"("Motion in"=w424, "Measurement Point"="height of stave", "Inital GO"=FALSE) -> ("Motion out"=w412:refnum<class "Motion.lvclass">, "Sum"=w413:dbl[])  [unwired: 4 in, 2 out]
          n132 = call "O to G v1.vi"("height"=w413, "south chip"=w414, "north chip"=w415, "Input file"=w416) -> ("output BR"=w419:dbl[], "output BL"=w417:dbl[], "output TL"=w418:dbl[])  [unwired: 5 in]
          "after NL" <- w418
          "after SR" <- w419
          n133 = Subtract(x=w419, y=w418) -> (x-y=w433:dbl[])
          n134 = Build Array(24.3 ("y"), 231.4 ("y"), 0.0 ("element"), -0.05 ("element")) -> ()  [unwired: 1 out]
          n135 = Subtract(x=w417, y=w418) -> (x-y=w439:dbl[])
          n136 = call "XY_to_Rotation_RPHI.vi"("X-Y"=w439) -> ("r-phi"=w438:dbl[])
          n137 = Index Array(array=w438, index=1) -> (element=w435:dbl)
          n138 = Multiply(x=w435, y=-1.0) -> (x*y=w429:dbl)
          n139 = Replace Array Subset(array=w433, new element=w429, index=3) -> (→"bless from OGP !! measured stave size  2":dbl[])
          n140 = Replace Array Subset(array=w418, new element=w429, index=3) -> (w431:dbl[])
          n141 = Add(x=w419, y=w418) -> (x+y=w445:dbl[])
          n142 = Divide(x=w445, y=2.0) -> (x/y=→"bless from OGP !!! Center of module on stave 3":dbl[])
        }
        n143 = Build Array(0.0 ("element"), 238.0 ("element"), 0.0 ("element"), 0.0 ("element")) -> (w378:dbl[])
        n144 = Add(x=w377, y=w378) -> (x+y=w376:dbl[])
        n145 = Build Array(w377, w376) -> (w375:dbl[][])
        n146 = Build Array(17.0 ("element"), 411.0 ("element"), 0.0 ("element"), 0.0 ("element")) -> (w388:dbl[])
        n147 = Build Array(17.0 ("element"), 60.9 ("element"), 0.0 ("element"), 0.0 ("element")) -> (w389:dbl[])
        n148 = case shown="True" w384 {
          tunnel: w389 -> [w464 w467]
          tunnel: w388 -> [w463 w466]
          tunnel: [w462 w465] -> w387
          frame False {
            n149 = Build Array(w463, w464) -> (w462:dbl[][])
          }
          frame True {
            n150 = Build Array(w467, w466) -> (w465:dbl[][])
          }
        }
        n151 = for {
          tunnel: w387 -> [w455] mode=indexing
          tunnel: w386 -> [w450]
          tunnel: w377 -> [w454]
          tunnel: [w452] -> w371 mode=indexing
          n152 = Multiply(x=w450, y=-1.0) -> (x*y=w449:dbl)
          n153 = Index Array(array=w455, index=0) -> (element=w458:dbl)
          n154 = Index Array(array=w455, index=1) -> (element=w457:dbl)
          n155 = call-poly <vilib>:"2D Cartesian Coordinate Rotation.vi"("theta"=w449, "y"=w457, "x"=w458) -> ("y out"=w460:dbl, "x out"=w459:dbl)  [unwired: 6 in, 1 out]
          n156 = Build Array(w459, w460, 0.0 ("element"), 0.0 ("element")) -> (w453:dbl[])
          n157 = Add(x=w453, y=w454) -> (x+y=w452:dbl[])
        }
        n158 = Add(x=w371, y=w370) -> (x+y=w369:dbl[][])
      }
      event "Measure Pickup Tools": Value Change {
        (unwired) "Measuring Pickup Tools" ("String")
        n159 = event-data() -> ()  [unwired: 1 in, 6 out]
        n160 = for {
          N: w470 -> [_]
          tunnel: [w503] -> w478 mode=indexing
          tunnel: w479 -> [w507]
          tunnel: [w489] -> w477
          tunnel: w476 -> [w488] mode=indexing
          # "Default size and\norientation"
          n161 = call "Joystick and Camera - external Connection.vi"("Motion in"=w507, "XYZTheta"=w488, "Measurement Point"="PickUp tool Top") -> ("Motion out"=w483:refnum<class "Motion.lvclass">, "Sum"=w506:dbl[])  [unwired: 4 in, 2 out]
          n162 = Build Array(0.0 ("element"), 29.94 ("element"), 0.0 ("element"), 0.0 ("element")) -> (w494:dbl[])
          n163 = Add(x=w506, y=w494) -> (x+y=w480:dbl[])
          n164 = Array Subset(array=w480, index=0, length=2) -> (w481:dbl[])
          n165 = call-dynamic "XY Go.vi"("Speed"=20.0, "XY"=w481, "Motion in"=w483) -> ("Motion out"=w482:refnum<class "Motion.lvclass">)  [unwired: 7 in, 1 out]
          n166 = call "Joystick and Camera - external Connection.vi"("Motion in"=w482, "Measurement Point"="PickUp tool Bottom", "Inital GO"=FALSE) -> ("Motion out"=w489:refnum<class "Motion.lvclass">, "Sum"=w505:dbl[])  [unwired: 4 in, 2 out]
          n167 = Add(x=w506, y=w505) -> (x+y=w512:dbl[])
          n168 = Subtract(x=w505, y=w506) -> (x-y=w504:dbl[])
          n169 = Divide(x=w512, y=2.0) -> (x/y=w509:dbl[])
          n170 = call "XYtoRPHI.vi"("X-Y"=w504) -> ("r-phi"=w510:dbl[])
          n171 = Index Array(array=w510, index=1) -> (element=w498:dbl)
          n172 = Absolute Value(x=w498) -> (abs(x)=w501:dbl)
          n173 = Sign(1:w498) -> (0:w499:dbl)
          n174 = Subtract(x=w501, y=1.5707963267948966) -> (x-y=w500:dbl)
          n175 = Multiply(x=w499, y=w500) -> (x*y=w497:dbl)
          n176 = Replace Array Subset(array=w509, new element=w497, index=3) -> (w503:dbl[])
          "PickupTool \nCenterPosition" <- w503
        }
      }
      event "Deposit Glue": Value Change {
        # "CF height"
        # "surface z offset"
        # "two sensor, Sensor B then A"
        # "Unmount syringe"
        # "first needle park position\nneedle gap on Z value : 0.5 mm"
        # "Syringe-camera offset"
        n177 = event-data() -> ()  [unwired: 1 in, 6 out]
        n178 = call-poly <vilib>:"Read Delimited Spreadsheet.vi"("file path (dialog if empty)"=path "D:/INTT/V1/Assembly Data/Tool Offsets/Dispense Tip Offset.txt", "number of rows (all:-1)"=-1) -> ("first row"=w568:dbl[])  [unwired: 8 in, 5 out]
        n179 = Add(x=14.2 ("element"), y=w524) -> (x+y=w518:dbl)
        n180 = Index Array(array=w568, index #1=0 ("index"), index #2=1 ("index")) -> (element #1=w563:dbl, element #2=w561:dbl)
        n181 = Build Array(w563, w561, 0.0 ("element"), 0.0 ("element")) -> (w547:dbl[])
        n182 = Array Subset(array=w514, index (row)=0, length (row)=1 ("length")) -> (w527:dbl[][])  [unwired: 2 in]
        n183 = Reshape Array(w527, 4 ("dimension size")) -> (w520:dbl[])
        n184 = Index Array(array=w520, index=2) -> (element=w515:dbl)
        n185 = Add(x=w515, y=w518) -> (x+y=w517:dbl)
        n186 = Build Array(436.638, 1040.76, w517, 0.0 ("element")) -> (w516:dbl[])
        "Needle parking position" <- w516
        n187 = call "XYZTheta Go.vi"("XYZTheta In"=w516, "Motion in"=w552) -> ("error out"=w560:errorcluster, "Motion out"=w551:refnum<class "Motion.lvclass">)  [unwired: 7 in, 1 out]
        n188 = call "Display Message to User"("error in (no error)"=w560) -> ("error out"=w553:errorcluster)  [unwired: 9 in, 1 out]
        n189 = case shown="False" w522 {
          tunnel: w514 -> [w576 w585]
          tunnel: [w573 w585] -> w521
          frame False {
            n190 = Array Subset(array=w576, index (row)=1 ("index"), length (row)=1 ("length")) -> (w577:dbl[][])  [unwired: 2 in]
            n191 = Array Subset(array=w576, index (row)=0 ("index"), length (row)=1 ("length")) -> (w580:dbl[][])  [unwired: 2 in]
            n192 = Reshape Array(w580, 4 ("dimension size")) -> (w575:dbl[])
            n193 = Reshape Array(w577, 4 ("dimension size")) -> (w574:dbl[])
            n194 = Build Array(w574, w575) -> (w573:dbl[][])
          }
          frame True {
          }
        }
        n195 = call-dynamic "Z Go.vi"("error in (no error)"=w553, "Speed"=20.0, "Position"=0.0, "Motion in"=w551) -> ("error out"=w550:errorcluster, "Motion out"=w556:refnum<class "Motion.lvclass">)  [unwired: 6 in]
        n196 = call "Display Message to User2"("error in (no error)"=w550) -> ("error out"=w549:errorcluster)  [unwired: 9 in, 1 out]
        n197 = Add(x=w515, y=-2.5) -> (x+y=w557:dbl)
        n198 = call-dynamic "Z Go.vi"("error in (no error)"=w549, "Speed"=20.0, "Position"=w557, "Motion in"=w556) -> ("error out"=w526:errorcluster, "Motion out"=w548:refnum<class "Motion.lvclass">)  [unwired: 6 in]
        n199 = call-dynamic "Connect.vi"("Ultimus V in"=refnum<class "Ultimus V2.lvclass"> refnum ("Ultimus V2.lvclass")) -> ("Ultimus V out"=w546:refnum<class "Ultimus V2.lvclass">)  [unwired: 9 in, 1 out]
        n200 = for {
          N: w541 -> [_]
          tunnel: w548 -> [w600]
          tunnel: w546 -> [w599]
          tunnel: w547 -> [w601]
          tunnel: w536 -> [_] mode=indexing
          tunnel: w521 -> [w602] mode=indexing
          tunnel: [w598] -> w534
          tunnel: [w597] -> w533
          tunnel: w526 -> [w593]
          tunnel: [w594] -> w525
          tunnel: w523 -> [w592]
          (unwired) 100.0 ("Speed")
          n201 = Add(x=w602, y=w601) -> (x+y=w632:dbl[])
          n202 = Add(x=w632, y=dbl[] [3.3, 5.0, 0.0, 0.0]) -> (x+y=w633:dbl[])
          n203 = Index Array(array=w633, index=2) -> (element=w590:dbl)
          n204 = Array Subset(array=w633, index=0, length=2) -> (w608:dbl[])
          n205 = call-dynamic "XY Go.vi"("error in (no error)"=w593, "Speed"=100.0, "XY"=w608, "Motion in"=w600) -> ("error out"=w588:errorcluster, "Motion out"=w589:refnum<class "Motion.lvclass">)  [unwired: 6 in]
          n206 = case shown="True" "check height?" {
            tunnel: w590 -> [_ w649]
            tunnel: w589 -> [w642 w648]
            tunnel: w588 -> [w643 w647]
            tunnel: [w643 w645] -> w587
            tunnel: [w642 w644] -> w586
            frame False {
            }
            frame True {
              n207 = call-dynamic "Z Go.vi"("error in (no error)"=w647, "Speed"=5.0, "Position"=w649, "Motion in"=w648) -> ("error out"=w646:errorcluster, "Motion out"=w644:refnum<class "Motion.lvclass">)  [unwired: 6 in]
              n208 = call "Display Message to User4"("error in (no error)"=w646) -> ("error out"=w645:errorcluster)  [unwired: 9 in, 1 out]
            }
          }
          n209 = Add(x=w590, y=-2.0) -> (x+y=w607:dbl)
          n210 = call-dynamic "Z Go.vi"("error in (no error)"=w587, "Speed"=5.0, "Position"=w607, "Motion in"=w586) -> ("error out"=w605:errorcluster, "Motion out"=w606:refnum<class "Motion.lvclass">)  [unwired: 6 in]
          n211 = call "Muliti_XY_dispense.vi"("Pressure"=w592, "Path count"=4, "distances"=dbl[][] [[0.0, 224.0], [27.4, 0.0], [0.0, -224.0], [-27.4, 0.0]], "Ultimus V in"=w599, "Motion in"=w606) -> ("Ultimus V out"=w626:refnum<class "Ultimus V2.lvclass">, "Motion out"=w631:refnum<class "Motion.lvclass">)  [unwired: 5 in]
          n212 = call-dynamic "wrtCurrent Go.vi"("axis names"=string[] ["X", "Y"], "error in (no error)"=w605, "Speed"=5.0, "distances"=dbl[] [4.6, 5.0], "Motion in"=w631) -> ("error out"=w596:errorcluster, "Motion out"=w625:refnum<class "Motion.lvclass">)  [unwired: 5 in]
          n213 = call "Muliti_XY_dispense.vi"("Pressure"=w592, "Path count"=4, "distances"=dbl[][] [[0.0, 214.0], [18.2, 0.0], [0.0, -214.0], [-18.2, 0.0]], "Ultimus V in"=w626, "Motion in"=w625) -> ("Ultimus V out"=w618:refnum<class "Ultimus V2.lvclass">, "Motion out"=w617:refnum<class "Motion.lvclass">)  [unwired: 5 in]
          n214 = call-dynamic "wrtCurrent Go.vi"("axis names"=string[] ["X", "Y"], "error in (no error)"=w596, "Speed"=5.0, "distances"=dbl[] [4.6, 5.0], "Motion in"=w617) -> ("error out"=w595:errorcluster, "Motion out"=w616:refnum<class "Motion.lvclass">)  [unwired: 5 in]
          n215 = call "Muliti_XY_dispense.vi"("Pressure"=w592, "Path count"=4, "distances"=dbl[][] [[0.0, 204.0], [9.0, 0.0], [0.0, -204.0], [-9.0, 0.0]], "Ultimus V in"=w618, "Motion in"=w616) -> ("Ultimus V out"=w603:refnum<class "Ultimus V2.lvclass">, "Motion out"=w604:refnum<class "Motion.lvclass">)  [unwired: 5 in]
          n216 = call-dynamic "wrtCurrent Go.vi"("axis names"=string[] ["X", "Y"], "error in (no error)"=w595, "Speed"=5.0, "distances"=dbl[] [4.5, 5.0], "Motion in"=w604) -> ("error out"=w594:errorcluster, "Motion out"=w610:refnum<class "Motion.lvclass">)  [unwired: 5 in]
          n217 = call "Muliti_XY_dispense.vi"("Pressure"=w592, "Path count"=1, "distances"=dbl[][] [[0.0, 194.0], [7.0, 0.0], [0.0, -206.0], [-7.0, 0.0]], "Ultimus V in"=w603, "Motion in"=w610) -> ("Ultimus V out"=w597:refnum<class "Ultimus V2.lvclass">, "Motion out"=w598:refnum<class "Motion.lvclass">)  [unwired: 5 in]
        }
        n218 = call "XYZTheta Go.vi"("error in (no error)"=w525, "XYZTheta In"=dbl[] [500.0, 1000.0, 0.0, 0.1], "Motion in"=w534) -> ("error out"=w544:errorcluster, "Motion out"=w542:refnum<class "Motion.lvclass">)  [unwired: 6 in, 1 out]
        n219 = call "Display Message to User3"("error in (no error)"=w544) -> ()  [unwired: 9 in, 2 out]
        n220 = call-dynamic "Disconnect.vi"("Ultimus V in"=w533) -> ()  [unwired: 9 in, 1 out]
      }
      event "Needle Alignment": Value Change {
        (unwired) "Needle Alignment in progress ...." ("String")
        # "CF height"
        # "surface z offset"
        # "first needle park position\nneedle gap on Z value : 0.5 mm"
        # "Syringe-camera offset"
        n221 = event-data() -> ()  [unwired: 1 in, 6 out]
        n222 = Array Subset(array=w652, index (row)=0, length (row)=1 ("length")) -> (w655:dbl[][])  [unwired: 2 in]
        n223 = Reshape Array(w655, 4 ("dimension size")) -> (w654:dbl[])
        n224 = Index Array(array=w654, index=2) -> (element=w651:dbl)
        n225 = call-poly <vilib>:"Read Delimited Spreadsheet.vi"("file path (dialog if empty)"=path "D:/INTT/V1/Assembly Data/Tool Offsets/Dispense Tip Offset.txt", "number of rows (all:-1)"=-1) -> ("first row"=w702:dbl[])  [unwired: 8 in, 5 out]
        n226 = Index Array(array=w702, index #1=0 ("index"), index #2=1 ("index")) -> (element #1=w697:dbl, element #2=w696:dbl)
        n227 = Add(x=14.2 ("element"), y=w660) -> (x+y=w662:dbl)
        n228 = Add(x=w651, y=w662) -> (x+y=w661:dbl)
        n229 = Build Array(436.638, 1040.76, w661, 0.0 ("element")) -> (w659:dbl[])
        n230 = Build Array(w697, w696, 0.0 ("element"), 0.0 ("element")) -> (w671:dbl[])
        n231 = call "XYZTheta Go.vi"("XYZTheta In"=w659, "Motion in"=w686) -> ("error out"=w695:errorcluster, "XYZTheta Out"=w676:dbl[], "Motion out"=w685:refnum<class "Motion.lvclass">)  [unwired: 7 in]
        n232 = call "Display Message to User10"("error in (no error)"=w695) -> ("error out"=w692:errorcluster)  [unwired: 9 in, 1 out]
        n233 = call-dynamic "Z Go.vi"("error in (no error)"=w692, "Speed"=20.0, "Position"=0.0, "Motion in"=w685) -> ("Motion out"=w684:refnum<class "Motion.lvclass">)  [unwired: 6 in, 1 out]
        n234 = Replace Array Subset(array=w676, new element=0.0 ("new element/subarray"), index=2) -> (w673:dbl[])
        n235 = call "Joystick and Camera - external Connection.vi"("Motion in"=w684, "XYZTheta"=w673, "Measurement Point"="Touch Needle on a surface") -> ("Motion out"=w682:refnum<class "Motion.lvclass">, "Gantry"=w672:dbl[])  [unwired: 4 in, 2 out]
        n236 = Subtract(x=w672, y=w671) -> (x-y=w670:dbl[])
        n237 = call "Joystick and Camera - external Connection.vi"("Motion in"=w682, "XYZTheta"=w670, "Measurement Point"="Measure the touch spot with camera") -> ("Motion out"=w678:refnum<class "Motion.lvclass">, "Gantry"=w681:dbl[])  [unwired: 4 in, 2 out]
        n238 = Subtract(x=w672, y=w681) -> (x-y=w680:dbl[])
        n239 = call-poly <vilib>:"Write Delimited Spreadsheet.vi"("file path (dialog if empty)"=path "D:/INTT/V1/Assembly Data/Tool Offsets/Dispense Tip Offset.txt", "1D data"=w680, "append to file? (new file:F)"=FALSE) -> ()  [unwired: 11 in, 2 out]
      }
      event "Pick and place": Value Change {
        (unwired) "PICK and PLACE samples ..." ("String")
        n240 = event-data() -> ()  [unwired: 1 in, 6 out]
        n241 = case shown="False" w706 {
          tunnel: w710 -> [w816 w838]
          tunnel: [w815 w837] -> w709
          frame False {
            n242 = Array Subset(array=w816, index (row)=0 ("index"), length (row)=1 ("length")) -> (w818:dbl[][])  [unwired: 2 in]
            n243 = Build Array(11.75 ("element"), 173.55 ("element"), 0.0 ("element"), 0.0 ("element")) -> (w822:dbl[])
            n244 = Reshape Array(w818, 4 ("dimension size")) -> (w817:dbl[])
            n245 = Add(x=w822, y=w817) -> (x+y=w815:dbl[])
          }
          frame True {
            n246 = Array Subset(array=w838, index (row)=0 ("index"), length (row)=1 ("length")) -> (w828:dbl[][])  [unwired: 2 in]
            n247 = Build Array(11.75 ("element"), 56.85 ("element"), 0.0 ("element"), 0.0 ("element")) -> (w832:dbl[])
            n248 = Reshape Array(w828, 4 ("dimension size")) -> (w827:dbl[])
            n249 = Add(x=w832, y=w827) -> (x+y=w837:dbl[])
          }
        }
        n250 = call-poly <vilib>:"Read Delimited Spreadsheet.vi"("file path (dialog if empty)"=path "D:/INTT/V1/Assembly Data/Tool Offsets/Bellows Tool Offset.txt", "number of rows (all:-1)"=-1) -> ("first row"=w727:dbl[])  [unwired: 8 in, 5 out]
        n251 = Index Array(array=w727, index #1=0 ("index"), index #2=1 ("index"), index #3=2 ("index")) -> (element #1=w723:dbl, element #2=w722:dbl, element #3=w721:dbl)
        n252 = for {
          N: 1 -> [_]
          tunnel: w730 -> [w736]
          tunnel: [w758] -> w720
          tunnel: w719 -> [w767] mode=indexing
          tunnel: [w745] -> w713
          tunnel: w714 -> [w735]
          tunnel: w723 -> [w760]
          tunnel: w722 -> [w759]
          tunnel: w721 -> [w757]
          tunnel: w715 -> [w751]
          tunnel: w712 -> [w738]
          tunnel: w709 -> [w737]
          tunnel: w707 -> [w733]
          w747 = 0 ("Write")
          w750 = TRUE ("Write Value")
          # "putback pickup tool"
          # "pickup tool"
          # "pickup tool height offset"
          # "Pick up PICKUP TOOL"
          # "Pick up CHIPs/Sensor and place on HDI"
          n253 = Build Array(w760, w759, w757, 0.0 ("element")) -> (w756:dbl[])
          n254 = Add(x=w767, y=w756) -> (x+y=w731:dbl[])
          n255 = call "XYZTheta-2Zspeed Go.vi"("XYZTheta In"=w731, "Motion in"=w736) -> ("error out"=w734:errorcluster, "Motion out"=w732:refnum<class "Motion.lvclass">)  [unwired: 7 in, 1 out]
          n256 = Replace Array Subset(array=w756, new element=-16.0 ("t"), index=2) -> (w754:dbl[])
          n257 = call "WriteReadWait.vi"("Read Value"=w750, "Write Value"=w750, "error in (no error)"=w734, "Read"=w747, "Write"=w747, "I-O in"=w735) -> ("error out"=w749:errorcluster, "I-O out"=w748:refnum<class "NI-DAQ.lvclass">)  [unwired: 4 in]
          n258 = for {
            N: w751 -> [_]
            tunnel: w732 -> [w779]
            tunnel: w754 -> [w778]
            tunnel: w749 -> [w777]
            tunnel: [w776] -> w761
            tunnel: w748 -> [w775]
            tunnel: [w774] -> w746
            tunnel: [w773] -> w753
            tunnel: w738 -> [w770]
            tunnel: w737 -> [w769]
            tunnel: w733 -> [w768] mode=indexing
            n259 = flat-sequence {
              tunnel: [w799] -> w780
              tunnel: w779 -> [w798]
              tunnel: w778 -> [w797]
              tunnel: w777 -> [w795]
              tunnel: w775 -> [w787]
              tunnel: [w794] -> w772
              tunnel: [w791] -> w771
              tunnel: w770 -> [w784]
              tunnel: w769 -> [w790]
              tunnel: w780 -> [w805]
              tunnel: [w814] -> w776
              tunnel: [w813] -> _
              tunnel: w778 -> [w807]
              tunnel: [w808] -> w774
              tunnel: [w803] -> w773
              tunnel: w772 -> [w810]
              tunnel: w771 -> [w804]
              tunnel: w768 -> [w806]
              frame #0 {
                w785 = FALSE ("Write Value")
                w792 = TRUE ("Write Value")
                w793 = 1 ("Write")
                # "pickup module"
                # "release module"
                # "pickup sample from tray"
                n260 = Add(x=w790, y=w797) -> (x+y=w796:dbl[])
                n261 = call "XYZTheta-2Zspeed Go.vi"("error in (no error)"=w795, "XYZTheta In"=w796, "Motion in"=w798) -> ("error out"=w788:errorcluster, "Motion out"=w799:refnum<class "Motion.lvclass">)  [unwired: 6 in, 1 out]
                n262 = call "Time Delay"("error in (no error)"=w788) -> ("error out"=w781:errorcluster)  [unwired: 10 in]
                n263 = call "?"("error in (no error)"=w781) -> ("error out"=w782:errorcluster)  [unwired: 9 in, 1 out]
                n264 = call "WriteReadWait.vi"("Read Value"=w785, "Write Value"=w785, "error in (no error)"=w782, "Read"=w784, "Write"=w784, "I-O in"=w787) -> ("error out"=w783:errorcluster, "I-O out"=w786:refnum<class "NI-DAQ.lvclass">)  [unwired: 4 in]
                n265 = call "Time Delay3"("error in (no error)"=w783) -> ("error out"=w789:errorcluster)  [unwired: 10 in]
                n266 = call "WriteReadWait.vi"("Read Value"=w792, "Write Value"=w792, "error in (no error)"=w789, "Read"=w793, "Write"=w793, "I-O in"=w786) -> ("error out"=w791:errorcluster, "I-O out"=w794:refnum<class "NI-DAQ.lvclass">)  [unwired: 4 in]
              }
              frame #1 {
                w809 = 1 ("Write")
                w811 = FALSE ("Write Value")
                # "lift for chip/sensor thickness"
                # "place sample on HDI"
                n267 = Add(x=w806, y=w807) -> (x+y=w802:dbl[])
                n268 = call "XYZTheta-2Zspeed Go.vi"("error in (no error)"=w804, "XYZTheta In"=w802, "Motion in"=w805) -> ("error out"=w801:errorcluster, "XYZTheta Out"=w813:dbl[], "Motion out"=w814:refnum<class "Motion.lvclass">)  [unwired: 6 in]
                n269 = call "1"("error in (no error)"=w801) -> ("error out"=w800:errorcluster)  [unwired: 9 in, 1 out]
                n270 = call "Time Delay6"("error in (no error)"=w800) -> ("error out"=w812:errorcluster)  [unwired: 10 in]
                n271 = call "WriteReadWait.vi"("Read Value"=w811, "Write Value"=w811, "error in (no error)"=w812, "Read"=w809, "Write"=w809, "I-O in"=w810) -> ("error out"=w803:errorcluster, "I-O out"=w808:refnum<class "NI-DAQ.lvclass">)  [unwired: 4 in]
              }
            }
          }
          n272 = call "XYZTheta-2Zspeed Go.vi"("error in (no error)"=w753, "XYZTheta In"=w731, "Motion in"=w761) -> ("error out"=w741:errorcluster, "Motion out"=w765:refnum<class "Motion.lvclass">)  [unwired: 6 in, 1 out]
          n273 = call "Time Delay9"("error in (no error)"=w741) -> ("error out"=w743:errorcluster)  [unwired: 10 in]
          n274 = call-dynamic "Digital Write 1 Channel.vi"("DAQ Module"=0, "error constant"=w743, "Value"=FALSE, "Channel"=0, "NI-DAQ.lvclass"=w746) -> ("error IO"=w742:errorcluster, "NI-DAQ.lvclass 2"=w745:refnum<class "NI-DAQ.lvclass">)  [unwired: 5 in]
          n275 = call "Time Delay10"("error in (no error)"=w742) -> ("error out"=w762:errorcluster)  [unwired: 10 in]
          n276 = call-dynamic "Z Go.vi"("error in (no error)"=w762, "Speed"=10.0, "Position"=0.0 ("new element/subarray"), "Motion in"=w765) -> ("Motion out"=w758:refnum<class "Motion.lvclass">)  [unwired: 6 in, 1 out]
        }
      }
      event "GOTO": Value Change {
        (unwired) "GOING to a position" ("String")
        n277 = event-data() -> ()  [unwired: 1 in, 6 out]
        n278 = call "XYZTheta Go.vi"("XYZTheta In"="Parking position", "Motion in"=w844) -> ("Motion out"=w842:refnum<class "Motion.lvclass">)  [unwired: 7 in, 2 out]
      }
      event "READ Position": Value Change {
        n279 = event-data() -> ()  [unwired: 1 in, 6 out]
        n280 = call-dynamic "Get Current Position.vi"("Motion in"=w862) -> ("XYZTheta Out"=→"Gantry current position":dbl[], "Motion out"=w861:refnum<class "Motion.lvclass">)  [unwired: 8 in, 1 out]
      }
      event "HDI vacuum": Value Change {
        n281 = event-data() -> ()  [unwired: 1 in, 6 out]
        n282 = call "WriteReadWait.vi"("Read Value"="vacuum", "Write Value"="vacuum", "Read"=w873, "Write"=w873, "I-O in"=w876) -> ("error out"=w874:errorcluster, "I-O out"=w863:refnum<class "NI-DAQ.lvclass">)  [unwired: 5 in]
        n283 = call "Time Delay2"("error in (no error)"=w874) -> ()  [unwired: 10 in, 1 out]
      }
      event Timeout {
        n284 = event-data() -> ()  [unwired: 1 in, 3 out]
        n285 = call-dynamic "Digital Read 1 Channel.vi"("Read"=w887, "NI-DAQ in"=w888) -> ("Value"=→"Status":bool, "NI-DAQ out"=w886:refnum<class "NI-DAQ.lvclass">)  [unwired: 7 in, 1 out]
      }
    }
    "Measured HDI size" <- w19
    "module position on stave" <- w20
    "Stave mark" <- w18
    "measured HDI top-left position" <- w15
    n286 = feedback-in #1(w19) -> ()
    n287 = feedback-in #2(w18) -> ()
    n288 = feedback-in #3(w15) -> ()
    n289 = feedback-in #4(w31) -> ()
    n290 = feedback-in #5(w28) -> ()
    n291 = feedback-in #6(w36) -> ()
    n292 = feedback-in #7(w20) -> ()
    n293 = feedback-in #8(w37) -> ()
    "# of tasks excuted" <- w33
  }
  n294 = call-dynamic "Disconnect.vi"("Controller in"=w4) -> ()  [unwired: 9 in, 1 out]
  n295 = call-dynamic "Disconnect.vi"("I-O in"=w1) -> ()  [unwired: 9 in, 1 out]
